vi "Velociprobe_Nanopositioner_Control_FPGA.vi"() -> ()   [LabVIEW 2015]
uses:
  <vilib>/Platform/TimedLoop/XDataNode/timing_clust.ctl
  <vilib>/Platform/TimedLoop/XDataNode/nitl_modes.ctl
  <vilib>/Platform/TimedLoop/XDataNode/wakeup.ctl
  Control X Up Down Ramp.ctl
  Control Y Up Down Ramp.ctl
  Detector_Trigger_Control.ctl
  <vilib>/rvi/Emulation/niFpgaSctlEmulationGetInTimedLoop.vi
  <vilib>/rvi/Emulation/niFpgaProcessEmulError.vi
  <vilib>/rvi/eio/common/nirviEmuTemplateMethod_errors.vi
  <vilib>/rvi/Emulation/niFpgaGetClockAttributes.vi
  <vilib>/rvi/Emulation/niFpgaEmulationReportErrorSimple.vi
  <vilib>/rvi/interface/RandomDataEmulation/niFpgaRandomDataHandleErrors.vi
  <vilib>/rvi/Emulation/niFpgaCriticalErrorInLSC.vi
  <vilib>/eio/EIONode/EIONode.xnode
  <vilib>/rvi/DataTransferAndStorage/Container/XNode/niFpgaContainer.xnode
  <vilib>/rvi/interface/RandomDataEmulation/nirviRandomDataFpgaReadWriteTemplate.vi
  <vilib>/rvi/Analysis/measure/butterworth/XNode/niFpgaButterworthFilter.xnode
  <vilib>/Platform/TimedLoop/XDataNode/XDataNode.xnode
  <vilib>/Platform/TimedLoop/XDataNode/XDNodeRunTimeDep.lvlib
panel:
  out "Number of Data Strings 2":i32
  out "Measured Data Trigger Time Period (Ticks)":u32
  in  "Data Trigger Time Period (uSec)":u32 caption="Detector Trigger Time Period (uSec)"
  out "Trigger for Data":fxp<+/-,58,25>
  out "Fly Scan Running":bool
  in  "Fly Scan Start":bool
  out "If True End Y Down Ramp":bool
  in  "Y Ramp Drop Size (nm)":fxp<+/-,16,16>
  out "Ramp Mid Range":bool
  out "If True End Up Ramp":bool
  out "Start or middle":bool=TRUE
  in  "Y Start Marker (nm)":fxp<+/-,58,25> format="%#_55g"
  out "Y Ramp Slope":fxp<+,48,16>
  in  "Y Ramp End (nm)":fxp<+/-,16,16>
  in  "Y Ramp Start (nm)":fxp<+/-,16,16>
  in  "Y Ramp Period (usec)":fxp<+,32,32>
  in  "X Ramp Period (usec)":fxp<+,32,32>
  in  "X Ramp End (nm)":fxp<+/-,16,16>
  in  "X Ramp Start (nm)":fxp<+/-,16,16>
  out "If True End X Down Ramp":bool
  out "X Ramp Mid Range":bool
  out "If True End X Up Ramp":bool
  out "Y Ramp Drop":bool
  out "Next Do Down Ramp":bool
  out "Continue Run":bool
  in  "X Start Marker (nm)":fxp<+/-,58,25>
  out "X Ramp Slope":fxp<+,48,16> format="%.37g"
  in  "DT Reset":bool
  in  "DT Duty Cycle (periods)":fxp<+,32,0>=0.5 caption="DT duty cycle (periods)"
  in  "DT Reference DC Offset (V)":fxp<+/-,16,16>
  in  "DT Reference Amplitude (V)":fxp<+/-,40,17>
  in  "DT Phase Offset (periods)":fxp<+,32,0>
  in  "DT Frequency (periods/tick)":fxp<+,32,0>=0.0002500000409781933
  in  "Trigger Wave Generator":T1(ring)
  out "If True End Trigger Low":bool
  in  "Trigger Low Level (V)":fxp<+/-,20,5>=-5.0
  in  "Trigger High Level (V)":fxp<+/-,20,5>=5.0
  out "If True End Trigger High":bool
  out "Trigger Mid High":bool
  in  "Trigger Low Period (usec)":fxp<+/-,64,45>
  in  "Trigger High Period (usec)":fxp<+/-,64,45>
  out "Measured Z Reference Time Period (Ticks)":u32
  in  "Z Reference Time Period (uSec)":u32
  in  "Z White Noise Amplitude":u16=32767
  in  "Z White Noise Seed":u32=4
  in  "Z Phase Offset (periods)":fxp<+,32,0>
  in  "Z Frequency (periods/tick)":fxp<+,32,0>=0.0002500000409781933
  in  "Z Reference DC Offset (nm)":fxp<+/-,16,16>
  in  "Z Reference Amplitude (nm)":fxp<+/-,40,17>
  in  "Z Reference Reset":bool
  in  "Z Reference Wave Selection":T2(ring)
  in  "Y White Noise Amplitude":u16=32767
  in  "Y White Noise Seed":u32=4
  out "Measured Y Reference Time Period (Ticks)":u32
  in  "Y Reference Time Period (uSec)":u32
  in  "Y Reference Reset":bool
  in  "Y Reference Wave Selection":T3(ring)
  in  "Detector Trigger Lower Limit (V)":fxp<+/-,20,5>=-5.0
  out "Detector Trigger In Range?":bool
  in  "Detector Trigger Upper Limit (V)":fxp<+/-,20,5>=5.0
  out "Detector Trigger (V)":fxp<+/-,20,5> format="%.29g"
  out "Measured Detector Trigger Time Period (Ticks)":u32
  in  "Detector Trigger Time Period (uSec)":u32
  out "Measured Trigger Gen Time Period (Ticks)":u32
  in  "Trigger Generation Time Period (uSec)":u32
  in  "Reference Signal Source":T4(ring)
  in  "Z-Stage Scaling Direction":fxp<+/-,3,3>=-1.0
  in  "Y-Stage Scaling Direction":fxp<+/-,3,3>=-1.0
  in  "Y Phase Offset (periods)":fxp<+,32,0>
  in  "Y Frequency (periods/tick)":fxp<+,32,0>=0.0002500000409781933
  in  "Optics and or Sample Stage":T5(ring)
  out "Z Stage External Reference (nm)":fxp<+/-,58,25>
  in  "Mod 3 AI2 V to nm Scaling":fxp<+,47,18>
  out "Mod 8 Input AI2 (V)":fxp<+/-,24,5>
  out "Y Stage External Reference (nm)":fxp<+/-,58,25>
  in  "Mod 3 AI1 V to nm Scaling":fxp<+,47,18>
  out "Mod 8 Input AI1 (V)":fxp<+/-,24,5>
  in  "Sample Z Stage Resolution (nm)":fxp<+,33,3>=0.001000046730041504
  in  "Sample Y Stage Resolution (nm)":fxp<+,33,3>=0.001000046730041504
  in  "Sample X Stage Resolution (nm)":fxp<+,33,3>=0.001000046730041504
  out "Sample Z Stage Displacement (nm)":fxp<+/-,58,25>
  out "Sample Z Stage Displacement raw (nm)":fxp<+/-,64,35> format="%.62g"
  out "Sample Y Stage Displacement (nm)":fxp<+/-,58,25>
  out "Sample Y Stage Displacement raw (nm)":fxp<+/-,64,35> format="%.41g"
  out "Sample X Stage Displacement raw (nm)":fxp<+/-,64,35> format="%.62g"
  out "Sample X Stage Displacement (nm)":fxp<+/-,58,25>
  in  "Reset Sample Z":bool
  out "32 bit Count Sample  Z":i32
  in  "Reset Sample Y":bool
  out "32 bit Count Sample  Y":i32
  in  "Reset Sample X":bool
  out "32 bit Count Sample X":i32
  out "Mod6/DIO3":bool
  out "Mod6/DIO2":bool
  out "Mod5/DIO3":bool
  out "Mod5/DIO2":bool
  out "Mod4/DIO3":bool
  out "Mod4/DIO2":bool
  out "Measured Analog Input Time Period (Ticks)":u32
  in  "Analog Input Time Period (uSec)":u32
  out "X Stage External Reference (nm)":fxp<+/-,58,25>
  in  "Mod 3 AI0 V to nm Scaling":fxp<+,47,18>
  out "Mod 3 Input AI0 (V)":fxp<+/-,24,5>
  out "Kxz Output, Kxz*ex (V)":fxp<+/-,58,25> format="%.31g"
  out "Kyz Output, Kyz*ey (V)":fxp<+/-,58,25> format="%.31g"
  in  "b02(2) yz1":fxp<+/-,64,9>[](array[numeric])=[0.0, 0.0, 0.0, 0.0, 0.0, 0.0, 0.0, 0.0, 0.0, 0.0, 0.0, 0.0, 0.0, 0.0, 0.0, 0.0, 0.0, 0.0, 0.0, 0.0]
  in  "b01(2) yz1":fxp<+/-,64,9>[](array[numeric])=[0.0, 0.0, 0.0, 0.0, 0.0, 0.0, 0.0, 0.0, 0.0, 0.0, 0.0, 0.0, 0.0, 0.0, 0.0, 0.0, 0.0, 0.0, 0.0, 0.0]
  in  "-a02(2) yz1":fxp<+/-,64,9>[](array[numeric])=[0.0, 0.0, 0.0, 0.0, 0.0, 0.0, 0.0, 0.0, 0.0, 0.0, 0.0, 0.0, 0.0, 0.0, 0.0, 0.0, 0.0, 0.0, 0.0, 0.0]
  in  "-a01(2) yz1":fxp<+/-,64,9>[](array[numeric])=[0.0, 0.0, 0.0, 0.0, 0.0, 0.0, 0.0, 0.0, 0.0, 0.0, 0.0, 0.0, 0.0, 0.0, 0.0, 0.0, 0.0, 0.0, 0.0, 0.0]
  in  "sos gain SF Controller yz1":fxp<+/-,42,9>
  in  "b02(2) xz1":fxp<+/-,64,9>[](array[numeric])=[0.0, 0.0, 0.0, 0.0, 0.0, 0.0, 0.0, 0.0, 0.0, 0.0, 0.0, 0.0, 0.0, 0.0, 0.0, 0.0, 0.0, 0.0, 0.0, 0.0]
  in  "b01(2) xz1":fxp<+/-,64,9>[](array[numeric])=[0.0, 0.0, 0.0, 0.0, 0.0, 0.0, 0.0, 0.0, 0.0, 0.0, 0.0, 0.0, 0.0, 0.0, 0.0, 0.0, 0.0, 0.0, 0.0, 0.0]
  in  "-a02(2) xz1":fxp<+/-,64,9>[](array[numeric])=[0.0, 0.0, 0.0, 0.0, 0.0, 0.0, 0.0, 0.0, 0.0, 0.0, 0.0, 0.0, 0.0, 0.0, 0.0, 0.0, 0.0, 0.0, 0.0, 0.0]
  in  "-a01(2) xz1":fxp<+/-,64,9>[](array[numeric])=[0.0, 0.0, 0.0, 0.0, 0.0, 0.0, 0.0, 0.0, 0.0, 0.0, 0.0, 0.0, 0.0, 0.0, 0.0, 0.0, 0.0, 0.0, 0.0, 0.0]
  in  "sos gain SF Controller xz1":fxp<+/-,42,9>
  out "Kzy Output, Kzy*ez (V)":fxp<+/-,58,25> format="%.31g"
  out "Kxy Output, Kxy*ex (V)":fxp<+/-,58,25> format="%.31g"
  in  "b02(2) zy1":fxp<+/-,64,9>[](array[numeric])=[0.0, 0.0, 0.0, 0.0, 0.0, 0.0, 0.0, 0.0, 0.0, 0.0, 0.0, 0.0, 0.0, 0.0, 0.0, 0.0, 0.0, 0.0, 0.0, 0.0]
  in  "b01(2) zy1":fxp<+/-,64,9>[](array[numeric])=[0.0, 0.0, 0.0, 0.0, 0.0, 0.0, 0.0, 0.0, 0.0, 0.0, 0.0, 0.0, 0.0, 0.0, 0.0, 0.0, 0.0, 0.0, 0.0, 0.0]
  in  "-a02(2) zy1":fxp<+/-,64,9>[](array[numeric])=[0.0, 0.0, 0.0, 0.0, 0.0, 0.0, 0.0, 0.0, 0.0, 0.0, 0.0, 0.0, 0.0, 0.0, 0.0, 0.0, 0.0, 0.0, 0.0, 0.0]
  in  "-a01(2) zy1":fxp<+/-,64,9>[](array[numeric])=[0.0, 0.0, 0.0, 0.0, 0.0, 0.0, 0.0, 0.0, 0.0, 0.0, 0.0, 0.0, 0.0, 0.0, 0.0, 0.0, 0.0, 0.0, 0.0, 0.0]
  in  "sos gain SF Controller zy1":fxp<+/-,42,9>
  in  "b02(2) xy1":fxp<+/-,64,9>[](array[numeric])=[0.0, 0.0, 0.0, 0.0, 0.0, 0.0, 0.0, 0.0, 0.0, 0.0, 0.0, 0.0, 0.0, 0.0, 0.0, 0.0, 0.0, 0.0, 0.0, 0.0]
  in  "b01(2) xy1":fxp<+/-,64,9>[](array[numeric])=[0.0, 0.0, 0.0, 0.0, 0.0, 0.0, 0.0, 0.0, 0.0, 0.0, 0.0, 0.0, 0.0, 0.0, 0.0, 0.0, 0.0, 0.0, 0.0, 0.0]
  in  "-a02(2) xy1":fxp<+/-,64,9>[](array[numeric])=[0.0, 0.0, 0.0, 0.0, 0.0, 0.0, 0.0, 0.0, 0.0, 0.0, 0.0, 0.0, 0.0, 0.0, 0.0, 0.0, 0.0, 0.0, 0.0, 0.0]
  in  "-a01(2) xy1":fxp<+/-,64,9>[](array[numeric])=[0.0, 0.0, 0.0, 0.0, 0.0, 0.0, 0.0, 0.0, 0.0, 0.0, 0.0, 0.0, 0.0, 0.0, 0.0, 0.0, 0.0, 0.0, 0.0, 0.0]
  in  "sos gain SF Controller xy1":fxp<+/-,42,9>
  out "Kzx Output, Kzx*ez (V)":fxp<+/-,58,25> format="%.31g"
  in  "b02(2) zx1":fxp<+/-,64,9>[](array[numeric])=[0.0, 0.0, 0.0, 0.0, 0.0, 0.0, 0.0, 0.0, 0.0, 0.0, 0.0, 0.0, 0.0, 0.0, 0.0, 0.0, 0.0, 0.0, 0.0, 0.0]
  in  "b01(2) zx1":fxp<+/-,64,9>[](array[numeric])=[0.0, 0.0, 0.0, 0.0, 0.0, 0.0, 0.0, 0.0, 0.0, 0.0, 0.0, 0.0, 0.0, 0.0, 0.0, 0.0, 0.0, 0.0, 0.0, 0.0]
  in  "-a02(2) zx1":fxp<+/-,64,9>[](array[numeric])=[0.0, 0.0, 0.0, 0.0, 0.0, 0.0, 0.0, 0.0, 0.0, 0.0, 0.0, 0.0, 0.0, 0.0, 0.0, 0.0, 0.0, 0.0, 0.0, 0.0]
  in  "-a01(2) zx1":fxp<+/-,64,9>[](array[numeric])=[0.0, 0.0, 0.0, 0.0, 0.0, 0.0, 0.0, 0.0, 0.0, 0.0, 0.0, 0.0, 0.0, 0.0, 0.0, 0.0, 0.0, 0.0, 0.0, 0.0]
  in  "sos gain SF Controller zx1":fxp<+/-,42,9>
  out "Kyx Output, Kyx*ey (V)":fxp<+/-,58,25> format="%.31g"
  in  "b02(2) yx1":fxp<+/-,64,9>[](array[numeric])=[0.0, 0.0, 0.0, 0.0, 0.0, 0.0, 0.0, 0.0, 0.0, 0.0, 0.0, 0.0, 0.0, 0.0, 0.0, 0.0, 0.0, 0.0, 0.0, 0.0]
  in  "b01(2) yx1":fxp<+/-,64,9>[](array[numeric])=[0.0, 0.0, 0.0, 0.0, 0.0, 0.0, 0.0, 0.0, 0.0, 0.0, 0.0, 0.0, 0.0, 0.0, 0.0, 0.0, 0.0, 0.0, 0.0, 0.0]
  in  "-a02(2) yx1":fxp<+/-,64,9>[](array[numeric])=[0.0, 0.0, 0.0, 0.0, 0.0, 0.0, 0.0, 0.0, 0.0, 0.0, 0.0, 0.0, 0.0, 0.0, 0.0, 0.0, 0.0, 0.0, 0.0, 0.0]
  in  "-a01(2) yx1":fxp<+/-,64,9>[](array[numeric])=[0.0, 0.0, 0.0, 0.0, 0.0, 0.0, 0.0, 0.0, 0.0, 0.0, 0.0, 0.0, 0.0, 0.0, 0.0, 0.0, 0.0, 0.0, 0.0, 0.0]
  in  "sos gain SF Controller yx1":fxp<+/-,42,9>
  in  "X-Stage Scaling Direction":fxp<+/-,3,3>=-1.0
  in  "Z-Stage nm to V Scaling":fxp<+/-,32,12>
  in  "Y-Stage nm to V Scaling":fxp<+/-,32,12>
  in  "X-Stage nm to V Scaling":fxp<+/-,32,12>
  out "Kxx Output, Kxx*ex (V)":fxp<+/-,58,25>
  out "Kyy Output, Kyy*ey (V)":fxp<+/-,58,25>
  out "Kzz Output, Kzz*ez (V)":fxp<+/-,58,25>
  in  "sos gain SF Controller xx1":fxp<+/-,42,9>
  in  "-a01(2) xx1":fxp<+/-,64,9>[](array[numeric])=[0.0, 0.0, 0.0, 0.0, 0.0, 0.0, 0.0, 0.0, 0.0, 0.0, 0.0, 0.0, 0.0, 0.0, 0.0, 0.0, 0.0, 0.0, 0.0, 0.0]
  in  "-a02(2) xx1":fxp<+/-,64,9>[](array[numeric])=[0.0, 0.0, 0.0, 0.0, 0.0, 0.0, 0.0, 0.0, 0.0, 0.0, 0.0, 0.0, 0.0, 0.0, 0.0, 0.0, 0.0, 0.0, 0.0, 0.0]
  in  "b01(2) xx1":fxp<+/-,64,9>[](array[numeric])=[0.0, 0.0, 0.0, 0.0, 0.0, 0.0, 0.0, 0.0, 0.0, 0.0, 0.0, 0.0, 0.0, 0.0, 0.0, 0.0, 0.0, 0.0, 0.0, 0.0]
  in  "b02(2) xx1":fxp<+/-,64,9>[](array[numeric])=[0.0, 0.0, 0.0, 0.0, 0.0, 0.0, 0.0, 0.0, 0.0, 0.0, 0.0, 0.0, 0.0, 0.0, 0.0, 0.0, 0.0, 0.0, 0.0, 0.0]
  in  "sos gain SF Controller yy1":fxp<+/-,42,9>
  in  "-a01(2) yy1":fxp<+/-,64,9>[](array[numeric])=[0.0, 0.0, 0.0, 0.0, 0.0, 0.0, 0.0, 0.0, 0.0, 0.0, 0.0, 0.0, 0.0, 0.0, 0.0, 0.0, 0.0, 0.0, 0.0, 0.0]
  in  "-a02(2) yy1":fxp<+/-,64,9>[](array[numeric])=[0.0, 0.0, 0.0, 0.0, 0.0, 0.0, 0.0, 0.0, 0.0, 0.0, 0.0, 0.0, 0.0, 0.0, 0.0, 0.0, 0.0, 0.0, 0.0, 0.0]
  in  "b01(2) yy1":fxp<+/-,64,9>[](array[numeric])=[0.0, 0.0, 0.0, 0.0, 0.0, 0.0, 0.0, 0.0, 0.0, 0.0, 0.0, 0.0, 0.0, 0.0, 0.0, 0.0, 0.0, 0.0, 0.0, 0.0]
  in  "b02(2) yy1":fxp<+/-,64,9>[](array[numeric])=[0.0, 0.0, 0.0, 0.0, 0.0, 0.0, 0.0, 0.0, 0.0, 0.0, 0.0, 0.0, 0.0, 0.0, 0.0, 0.0, 0.0, 0.0, 0.0, 0.0]
  in  "sos gain SF Controller zz1":fxp<+/-,42,9>
  in  "-a01(2) zz1":fxp<+/-,64,9>[](array[numeric])=[0.0, 0.0, 0.0, 0.0, 0.0, 0.0, 0.0, 0.0, 0.0, 0.0, 0.0, 0.0, 0.0, 0.0, 0.0, 0.0, 0.0, 0.0, 0.0, 0.0]
  in  "-a02(2) zz1":fxp<+/-,64,9>[](array[numeric])=[0.0, 0.0, 0.0, 0.0, 0.0, 0.0, 0.0, 0.0, 0.0, 0.0, 0.0, 0.0, 0.0, 0.0, 0.0, 0.0, 0.0, 0.0, 0.0, 0.0]
  in  "b01(2) zz1":fxp<+/-,64,9>[](array[numeric])=[0.0, 0.0, 0.0, 0.0, 0.0, 0.0, 0.0, 0.0, 0.0, 0.0, 0.0, 0.0, 0.0, 0.0, 0.0, 0.0, 0.0, 0.0, 0.0, 0.0]
  in  "b02(2) zz1":fxp<+/-,64,9>[](array[numeric])=[0.0, 0.0, 0.0, 0.0, 0.0, 0.0, 0.0, 0.0, 0.0, 0.0, 0.0, 0.0, 0.0, 0.0, 0.0, 0.0, 0.0, 0.0, 0.0, 0.0]
  in  "Scaling mV to V":fxp<+,33,10>=0.0009765625
  in  "System Loop Type":enum16{"Open Loop", "Closed Loop"}(ring)
  in  "Timeout FPGA FIFO1":i32=40000000
  out "FIFO Timed Out":bool
  in  "Interrupt Boolean":bool
  out "Wait Until Cleared":bool
  out "Number of Data Strings":i32
  in  "Y Reference DC Offset (nm)":fxp<+/-,16,16>
  in  "X Reference DC Offset (nm)":fxp<+/-,16,16>
  in  "Y Reference Amplitude (nm)":fxp<+/-,40,17>
  out "Z Stage Reference (nm)":fxp<+/-,58,25> format="%.41g"
  out "Y Stage Reference (nm)":fxp<+/-,58,25> format="%.41g"
  out "Optics Z Stage Displacement (nm)":fxp<+/-,58,25>
  out "Optics Z Stage Displacement raw (nm)":fxp<+/-,64,35>
  in  "Optics Z Stage Resolution (nm)":fxp<+,33,3>=0.001000046730041504
  in  "Reset Optics Z":bool
  out "32 bit Count Optics  Z":i32
  out "Mod6/DIO1":bool
  out "Mod6/DIO0":bool
  out "Optics Y Stage Displacement (nm)":fxp<+/-,58,25>
  out "Optics Y Stage Displacement raw (nm)":fxp<+/-,64,35>
  in  "Optics Y Stage Resolution (nm)":fxp<+,33,3>=0.001000046730041504
  in  "Reset Optics Y":bool
  out "32 bit Count Optics  Y":i32
  out "Mod5/DIO1":bool
  out "Mod5/DIO0":bool
  out "Z-Stage Input In Range?":bool
  out "Y-Stage Input In Range?":bool
  in  "Controller Output Lower Limit":fxp<+/-,20,5>=-5.0
  out "X-Stage Input In Range?":bool
  in  "Controller Output Upper Limit":fxp<+/-,20,5>=5.0
  in  "X White Noise Amplitude":u16=32767
  in  "X White Noise Seed":u32=4
  in  "X Reference Reset":bool
  in  "X Reference Wave Selection":T6(ring)
  out "Measured Counter Time Period (Ticks)":u32
  out "Measured Datalog Time Period (Ticks)":u32
  out "Measured Plant Output Time Period (Ticks)":u32
  out "Measured Controller Output Time Period (Ticks)":u32
  out "Measured Controller Time Period (Ticks)":u32
  out "Measured X Reference Time Period (Ticks)":u32
  out "Optics X Stage Displacement raw (nm)":fxp<+/-,64,35>
  in  "Optics X Stage Resolution (nm)":fxp<+,33,3>=0.001000046730041504 format="%#_31g"
  in  "Plant Output Time Period (uSec)":u32
  out "Optics X Stage Displacement (nm)":fxp<+/-,58,25>
  in  "Reset Optics X":bool
  out "32 bit Count Optics X":i32
  out "Mod4/DIO1":bool
  out "Mod4/DIO0":bool
  out "error out (FPGA)":errorcluster
  out "error out (AO FPGA)":errorcluster
  out "stop case":bool
  in  "Controller Output Time Period (uSec)":u32
  in  "Datalog Cases":T7(ring)
  out "PI Z-Stage Input (V)":fxp<+/-,20,5> format="%.29g"
  out "PI Y-Stage Input (V)":fxp<+/-,20,5> format="%.29g"
  out "PI X-Stage Input (V)":fxp<+/-,20,5> format="%.29g"
  in  "Controller Time Period (uSec)":u32
  in  "Datalog Time Period (uSec)":u32
  in  "X Reference Time Period (uSec)":u32
  in  "X Reference Amplitude (nm)":fxp<+/-,40,17>
  out "X Stage Reference (nm)":fxp<+/-,58,25> format="%.41g"
  out "FIFO Timed Out?":bool
  in  "X Phase Offset (periods)":fxp<+,32,0>
  in  "X Frequency (periods/tick)":fxp<+,32,0>=0.0002500000409781933
types:
  T1 = enum16{"Custom Square Wave ", "Square Wave 1", "Square Wave 2"}
  T2 = enum16{"Constant", "Sine Wave", "Sawtooth Wave", "Square Wave", "Filtered White Noise"}
  T3 = enum16{"Constant", "Sine Wave", "Custom Ramp Wave", "Filtered White Noise"}
  T4 = enum16{"FPGA Generated Reference", "External Reference"}
  T5 = enum16{"Optics Stage Only", "Optics and Sample Stage"}
  T6 = enum16{"Constant", "Sine Wave", "Custom Up Down Ramp", "Filtered White Noise"}
  T7 = enum16{"Data Log 1", "Data Log 2", "Data Log 3", "Data Log 4", "Data Log 5", "Data Log 6", "Data Log 7", "Data Log 8", "Data Log 9", "Data Log 10", "Data Log 11", "Data Log 12", "Data Log 13", "Data Log 14", "Data Log 15", "Data Log 16"}
  T8 = typedef "Control Y Up Down Ramp.ctl" = enum16{"Y Up Ramp", "Y Down Ramp"}
  T9 = typedef "Detector_Trigger_Control.ctl" = enum16{"Trigger High", "Trigger Low"}
  T10 = typedef "XDNodeRunTimeDep.lvlib/timing_clust.ctl" = cluster{"Expected End [f-1]":u64, "Actual End [f-1]":u64, "Finished Late? [f-1]":bool, "Expected End [i-1]":u64, "Actual End [i-1]":u64, "Finished Late? [i-1]":bool, "Expected Start [i]":u64, "Actual Start [i]":u64, "Expected Start [f]":u64, "Actual Start [f]":u64, "Source Name":string, "Structure Name":string, "Period":i64, "Deadline":i64, "Offset":i64, "Start":i64, "Priority":i32, "Timeout":i32, "Mode":T11, "Wakeup Reason":T12, "Error":errorcluster, "Source Type":string, "Secondary Source Type":string, "Global End Time":u64, "Global Start Time":u64, "Frame Duration":u64, "Iteration Duration":u64, "Assigned CPU":i32, "I/O Scan Engine Mode":u32}
  T11 = typedef "XDNodeRunTimeDep.lvlib/nitl_modes.ctl" = enum32{"No Change", "Process missed periods, maintain original phase", "Discard missed periods, maintain original phase", "Process missed periods, ignore original phase", "Discard missed periods, ignore original phase"}
  T12 = typedef "XDNodeRunTimeDep.lvlib/wakeup.ctl" = enum32{"Normal", "Aborted", "Asynchronous wakeup", "Timing source error", "Timed loop error", "Timeout"}
  T13 = typedef "Control X Up Down Ramp.ctl" = enum16{"X Up Ramp", "X Down Ramp"}
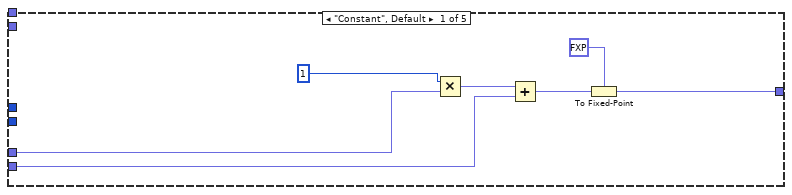
[diagram p2: hidden frame]
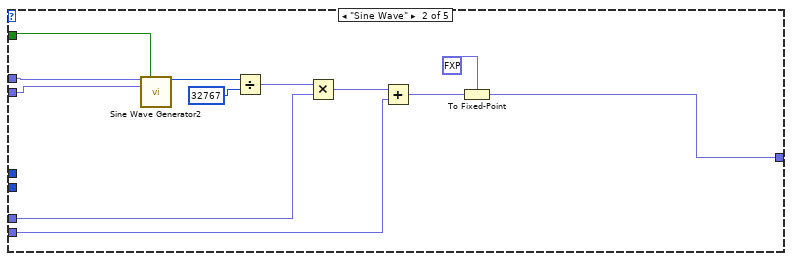
[diagram p3: hidden frame]
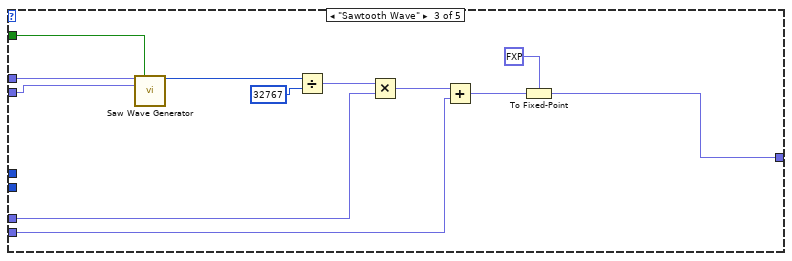
[diagram p4: hidden frame]
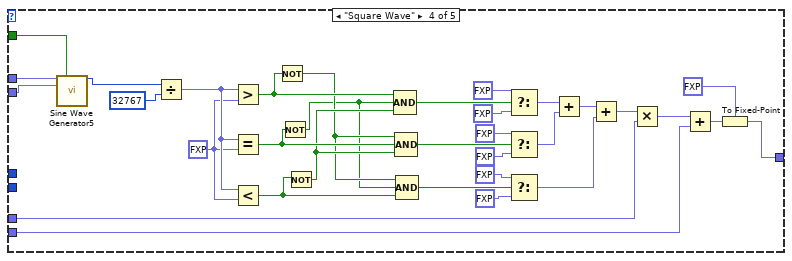
[diagram p5: hidden frame]
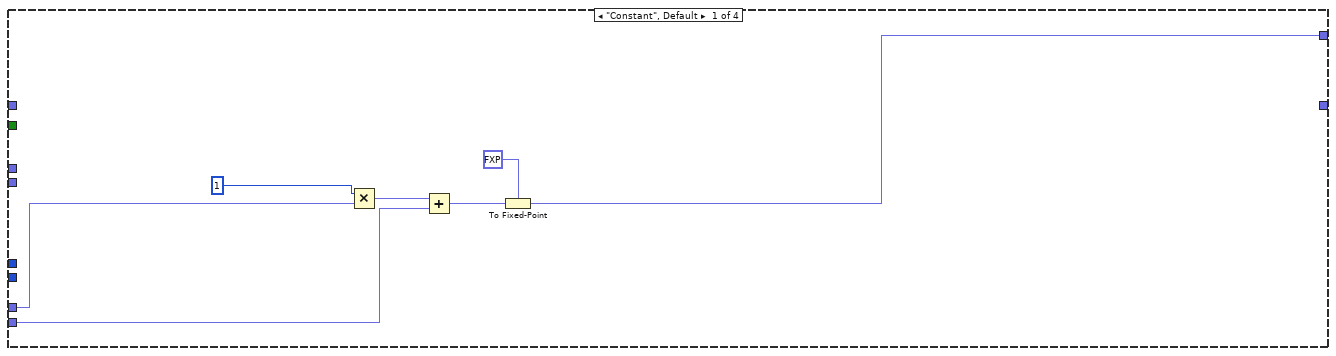
[diagram p6: hidden frame]
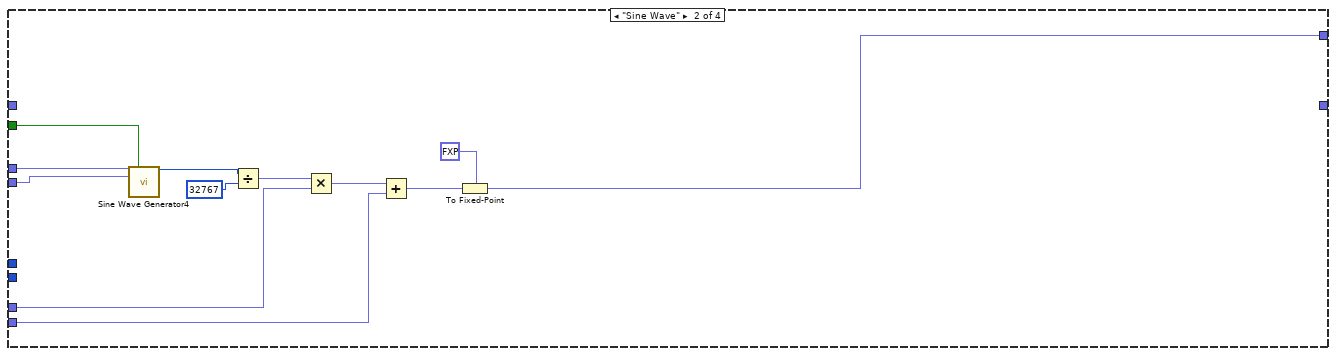
[diagram p7: hidden frame]
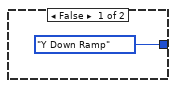
[diagram p8: hidden frame]
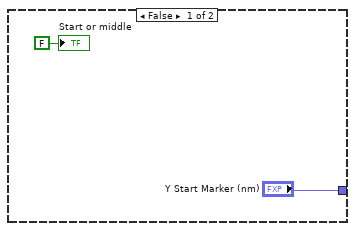
[diagram p9: hidden frame]
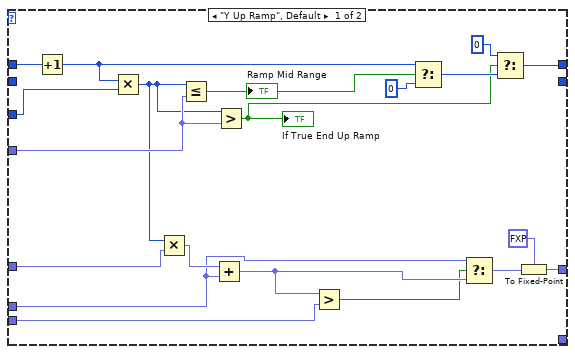
[diagram p10: hidden frame]
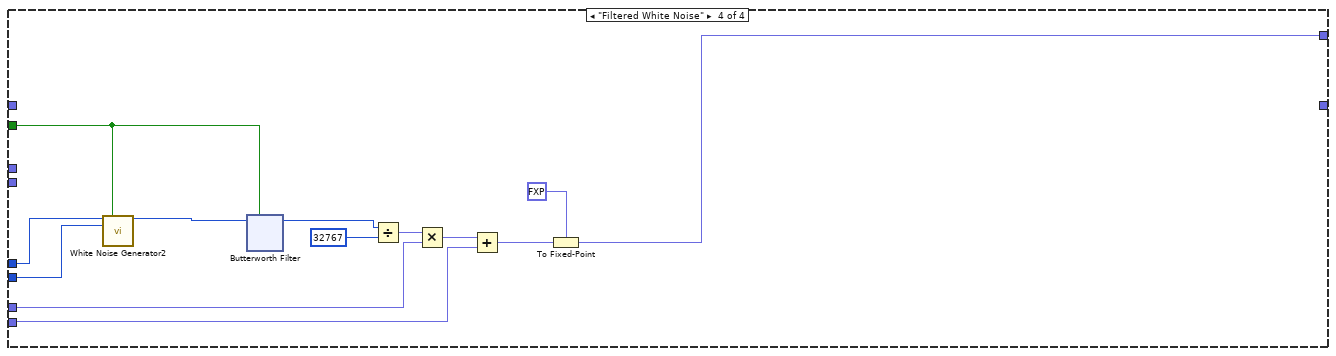
[diagram p13: hidden frame]
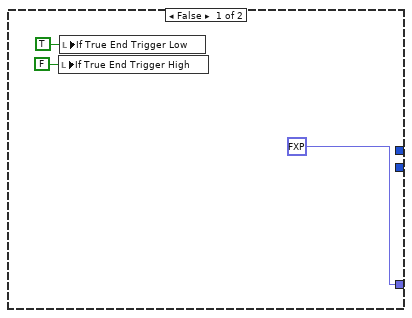
[diagram p14: hidden frame]
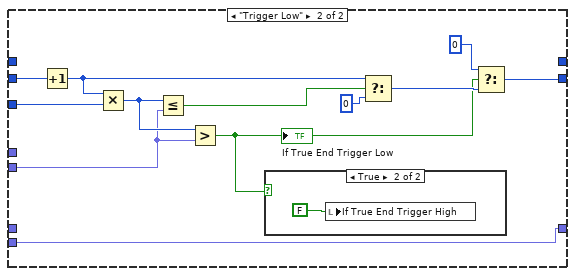
[diagram p16: hidden frame]
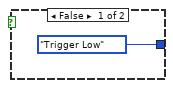
[diagram p18: hidden frame]
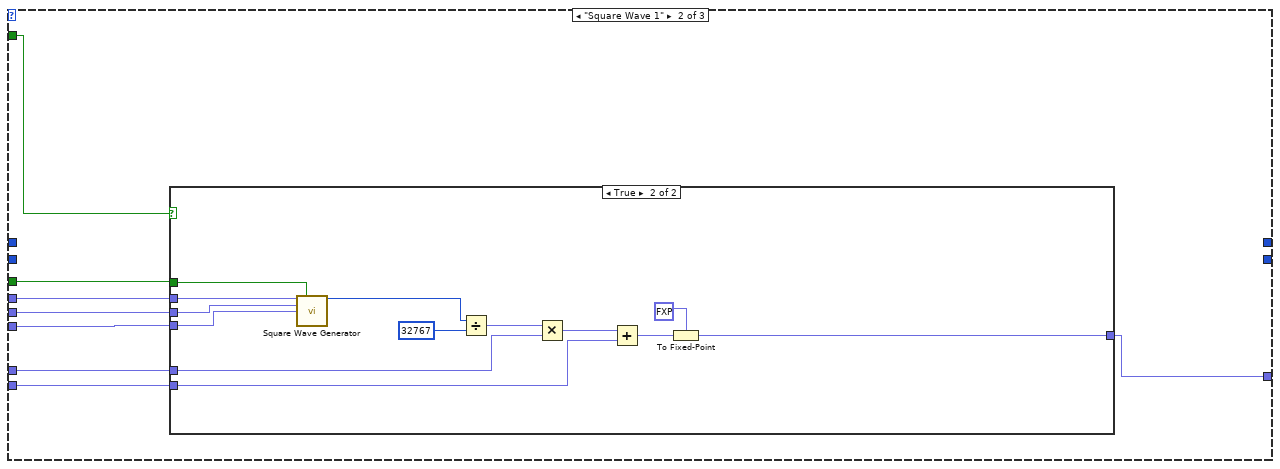
[diagram p19: hidden frame]
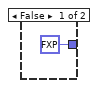
[diagram p20: hidden frame]
diagram:
  n1 = flat-sequence {
    tunnel: [w4] -> w1
    tunnel: [w10] -> w3
    tunnel: w1 -> [w10]
    frame #0 {
      n2 = xnode "FPGA I/O Node"("Mod3/Start"=TRUE ("I/O Item")) -> ("error out"=w4:errorcluster)  [unwired: 2 in, 1 out]
      "error out (AO FPGA)" <- w4
      "stop case" <- FALSE ("stop case")
    }
    frame #1 {
      w9 = u8 0  # IRQ Number (0)
      n3 = Not(x="Interrupt Boolean") -> (.not. x?=w7:bool)
      "Wait Until Cleared" <- w7
      n4 = call <vilib>:"niFPGA Interrupt.vi"("Wait Until Cleared (F)"=w7, "IRQ Number (0)"=w9) -> ()  [unwired: 1 in]
    }
  }
  n5 = case shown="No Error" w3 {
    selector: w3 -> [_ w1943]
    tunnel: [w30 w1943] -> w2
    frame No Error {
      w21 = errorcluster {"status"=FALSE, "code"=0, "source"=""}  # Error
      w15 = 0
      n6 = while {
        tunnel: [w1554] -> w24
        shift-right: [w1547] -> _
        shift-left: _ -> [w1546]
        shift-right: [w1543] -> _
        shift-left: _ -> [w1542]
        stop <- w1552 stop-if-true
        n7 = local read "Detector Trigger (V)"() -> (w1547:fxp<+/-,20,5>)
        n8 = local read "Trigger for Data"() -> (w1543:fxp<+/-,58,25>)
        n9 = local read "Fly Scan Running"() -> (w1544:bool)
        n10 = Greater?(x=w1547, y=w1546) -> (0:w1545:bool)
        n11 = Greater?(x=w1543, y=w1542) -> (0:w1541:bool)
        n12 = case shown="True" w1544 {
          tunnel: [w1558 w1571] -> w1555
          tunnel: [w1559 w1570] -> w1548
          tunnel: w1545 -> [_ w1569]
          tunnel: w1541 -> [w1557 _]
          frame False {
            w1566 = 5  # # of Data Strings
            n13 = case shown="True" w1557 {
              tunnel: w1566 -> [_ w1567]
              tunnel: fxp<+/-,58,25> 0.0 ("fixed-point type") -> [_ w1568]
              tunnel: [_ w1568] -> w1564
              tunnel: [_ w1568] -> w1562
              tunnel: [_ w1568] -> w1561
              tunnel: [_ w1568] -> w1560
              tunnel: [_ w1568] -> w1563
              tunnel: [_ w1567] -> w1558
              frame False {
              }
              frame True {
              }
            }
            "Number of Data Strings 2" <- w1558
            n14 = Build Array "Build Array"(w1564, w1563, w1562, w1561, w1560) -> (w1559:fxp<+/-,58,25>[])
          }
          frame True {
            n15 = case shown="True" w1569 {
              tunnel: [_ w1578] -> w1571
              tunnel: [_ w1574] -> w1570
              frame False {
              }
              frame True {
                w1579 = 5  # # of Data Strings
                n16 = local read "Sample X Stage Displacement (nm)"() -> (w1585:fxp<+/-,58,25>)
                n17 = local read "Sample Y Stage Displacement (nm)"() -> (w1584:fxp<+/-,58,25>)
                n18 = local read "Sample Z Stage Displacement (nm)"() -> (w1583:fxp<+/-,58,25>)
                n19 = local read "Optics X Stage Displacement (nm)"() -> (w1589:fxp<+/-,58,25>)
                n20 = local read "Optics Y Stage Displacement (nm)"() -> (w1588:fxp<+/-,58,25>)
                n21 = local read "Optics Z Stage Displacement (nm)"() -> (w1586:fxp<+/-,58,25>)
                n22 = local read "X Stage External Reference (nm)"() -> (w1577:fxp<+/-,58,25>)
                n23 = local read "Y Stage External Reference (nm)"() -> (w1576:fxp<+/-,58,25>)
                n24 = local read "Z Stage External Reference (nm)"() -> (w1575:fxp<+/-,58,25>)
                n25 = local read "X Stage Reference (nm)"() -> (w1597:fxp<+/-,58,25>)
                n26 = local read "Y Stage Reference (nm)"() -> (w1582:fxp<+/-,58,25>)
                n27 = local read "Z Stage Reference (nm)"() -> (w1581:fxp<+/-,58,25>)
                n28 = local read "Detector Trigger (V)"() -> (w1573:fxp<+/-,20,5>)
                n29 = local read "PI X-Stage Input (V)"() -> (w1596:fxp<+/-,20,5>)
                n30 = local read "PI Y-Stage Input (V)"() -> (w1595:fxp<+/-,20,5>)
                n31 = local read "PI Z-Stage Input (V)"() -> (w1594:fxp<+/-,20,5>)
                n32 = case shown="\"Data Log 16\"" "Datalog Cases" {
                  tunnel: fxp<+/-,58,25> 0.0 ("fixed-point type") -> [w1599 w1612 w1621 w1634 w1643 w1658 w1671 w1683 w1701 w1713 w1723 w1735 w1746 w1758 w1769 w1781]
                  tunnel: [w1608 w1619 w1631 w1642 w1655 w1668 w1678 w1695 w1705 w1719 w1728 w1743 w1755 w1766 w1777 w1789] -> w1592
                  tunnel: w1597 -> [w1609 _ _ _ w1648 _ _ _ _ _ _ _ _ _ _ w1785]
                  tunnel: w1596 -> [w1605 _ _ _ w1647 _ _ _ _ w1720 _ _ w1750 _ _ _]
                  tunnel: w1595 -> [_ w1618 _ _ _ w1662 _ _ _ _ w1733 _ _ w1761 _ _]
                  tunnel: w1594 -> [_ _ w1628 _ _ _ w1675 _ _ _ _ w1744 _ _ w1772 _]
                  tunnel: [w1607 w1611 w1630 w1636 w1654 w1667 w1677 w1691 w1704 w1714 w1727 w1742 w1754 w1765 w1776 w1788] -> w1591
                  tunnel: [w1606 w1620 w1629 w1641 w1653 w1666 w1676 w1687 w1703 w1715 w1726 w1741 w1753 w1764 w1775 w1787] -> w1590
                  tunnel: w1589 -> [w1602 _ _ w1638 w1650 _ _ w1698 _ w1718 w1732 w1739 w1749 _ _ w1783]
                  tunnel: w1588 -> [_ w1614 _ w1637 _ w1661 _ w1694 _ w1717 w1731 w1738 _ w1760 _ w1782]
                  tunnel: fxp<+/-,40,17> 0.0 ("fixed-point type") -> [w1601 w1613 w1623 w1632 w1645 w1657 w1669 w1682 w1699 w1710 w1722 w1734 w1748 w1757 w1768 _]
                  tunnel: w1586 -> [_ _ w1624 w1635 _ _ w1674 w1690 _ w1711 w1730 w1737 _ _ w1771 _]
                  tunnel: w1585 -> [_ _ _ _ w1649 _ _ w1697 w1708 _ _ _ _ _ _ _]
                  tunnel: w1584 -> [_ _ _ _ _ w1660 _ w1693 w1707 _ _ _ _ _ _ _]
                  tunnel: w1583 -> [_ _ _ _ _ _ w1673 w1689 w1706 _ _ _ _ _ _ _]
                  tunnel: w1582 -> [_ w1617 _ _ _ w1663 _ _ _ _ _ _ _ _ _ w1784]
                  tunnel: w1581 -> [_ _ w1627 _ _ _ w1679 _ _ _ _ _ _ _ _ _]
                  tunnel: [w1604 w1616 w1626 w1640 w1652 w1665 w1672 w1686 w1702 w1716 w1725 w1740 w1752 w1763 w1774 w1786] -> w1580
                  tunnel: w1579 -> [w1603 w1615 w1625 w1639 w1651 w1664 w1680 w1685 w1709 w1721 w1729 w1745 w1756 w1767 w1778 w1790]
                  tunnel: [w1603 w1615 w1625 w1639 w1651 w1664 w1680 w1685 w1709 w1721 w1729 w1745 w1756 w1767 w1778 w1790] -> w1578
                  tunnel: w1577 -> [_ _ _ _ _ _ _ _ _ _ _ _ w1751 _ _ _]
                  tunnel: w1576 -> [_ _ _ _ _ _ _ _ _ _ _ _ _ w1762 _ _]
                  tunnel: w1575 -> [_ _ _ _ _ _ _ _ _ _ _ _ _ _ w1773 _]
                  tunnel: w1573 -> [_ _ _ _ _ _ _ _ _ _ _ _ _ _ _ w1780]
                  tunnel: [w1600 w1610 w1622 w1633 w1644 w1656 w1670 w1684 w1700 w1712 w1724 w1736 w1747 w1759 w1770 w1779] -> w1572
                  frame "Data Log 1", Default {
                    n33 = To Fixed-Point(fixed-point type=w1599, number=w1609) -> (fixed-point=w1608:fxp<+/-,58,25>)
                    n34 = To Fixed-Point(fixed-point type=w1599, number=w1605) -> (fixed-point=w1607:fxp<+/-,58,25>)
                    n35 = To Fixed-Point(fixed-point type=w1599, number=w1602) -> (fixed-point=w1606:fxp<+/-,58,25>)
                    n36 = To Fixed-Point(fixed-point type=w1599, number=w1601) -> (fixed-point=w1604:fxp<+/-,58,25>)
                    n37 = To Fixed-Point(fixed-point type=w1599, number=w1601) -> (fixed-point=w1600:fxp<+/-,58,25>)
                  }
                  frame "Data Log 2" {
                    n38 = To Fixed-Point(fixed-point type=w1612, number=w1617) -> (fixed-point=w1619:fxp<+/-,58,25>)
                    n39 = To Fixed-Point(fixed-point type=w1612, number=w1618) -> (fixed-point=w1611:fxp<+/-,58,25>)
                    n40 = To Fixed-Point(fixed-point type=w1612, number=w1614) -> (fixed-point=w1620:fxp<+/-,58,25>)
                    n41 = To Fixed-Point(fixed-point type=w1612, number=w1613) -> (fixed-point=w1616:fxp<+/-,58,25>)
                    n42 = To Fixed-Point(fixed-point type=w1612, number=w1613) -> (fixed-point=w1610:fxp<+/-,58,25>)
                  }
                  frame "Data Log 3" {
                    n43 = To Fixed-Point(fixed-point type=w1621, number=w1627) -> (fixed-point=w1631:fxp<+/-,58,25>)
                    n44 = To Fixed-Point(fixed-point type=w1621, number=w1628) -> (fixed-point=w1630:fxp<+/-,58,25>)
                    n45 = To Fixed-Point(fixed-point type=w1621, number=w1624) -> (fixed-point=w1629:fxp<+/-,58,25>)
                    n46 = To Fixed-Point(fixed-point type=w1621, number=w1623) -> (fixed-point=w1626:fxp<+/-,58,25>)
                    n47 = To Fixed-Point(fixed-point type=w1621, number=w1623) -> (fixed-point=w1622:fxp<+/-,58,25>)
                  }
                  frame "Data Log 4" {
                    n48 = To Fixed-Point(fixed-point type=w1634, number=w1638) -> (fixed-point=w1642:fxp<+/-,58,25>)
                    n49 = To Fixed-Point(fixed-point type=w1634, number=w1637) -> (fixed-point=w1636:fxp<+/-,58,25>)
                    n50 = To Fixed-Point(fixed-point type=w1634, number=w1635) -> (fixed-point=w1641:fxp<+/-,58,25>)
                    n51 = To Fixed-Point(fixed-point type=w1634, number=w1632) -> (fixed-point=w1640:fxp<+/-,58,25>)
                    n52 = To Fixed-Point(fixed-point type=w1634, number=w1632) -> (fixed-point=w1633:fxp<+/-,58,25>)
                  }
                  frame "Data Log 5" {
                    n53 = To Fixed-Point(fixed-point type=w1643, number=w1648) -> (fixed-point=w1655:fxp<+/-,58,25>)
                    n54 = Subtract(x=w1650, y=w1649) -> (x-y=w1646:fxp<+/-,59,26>)
                    n55 = To Fixed-Point(fixed-point type=w1643, number=w1647) -> (fixed-point=w1654:fxp<+/-,58,25>)
                    n56 = To Fixed-Point(fixed-point type=w1643, number=w1646) -> (fixed-point=w1653:fxp<+/-,58,25>)
                    n57 = To Fixed-Point(fixed-point type=w1643, number=w1645) -> (fixed-point=w1652:fxp<+/-,58,25>)
                    n58 = To Fixed-Point(fixed-point type=w1643, number=w1645) -> (fixed-point=w1644:fxp<+/-,58,25>)
                  }
                  frame "Data Log 6" {
                    n59 = To Fixed-Point(fixed-point type=w1658, number=w1663) -> (fixed-point=w1668:fxp<+/-,58,25>)
                    n60 = To Fixed-Point(fixed-point type=w1658, number=w1662) -> (fixed-point=w1667:fxp<+/-,58,25>)
                    n61 = Subtract(x=w1661, y=w1660) -> (x-y=w1659:fxp<+/-,59,26>)
                    n62 = To Fixed-Point(fixed-point type=w1658, number=w1659) -> (fixed-point=w1666:fxp<+/-,58,25>)
                    n63 = To Fixed-Point(fixed-point type=w1658, number=w1657) -> (fixed-point=w1665:fxp<+/-,58,25>)
                    n64 = To Fixed-Point(fixed-point type=w1658, number=w1657) -> (fixed-point=w1656:fxp<+/-,58,25>)
                  }
                  frame "Data Log 7" {
                    n65 = To Fixed-Point(fixed-point type=w1671, number=w1679) -> (fixed-point=w1678:fxp<+/-,58,25>)
                    n66 = To Fixed-Point(fixed-point type=w1671, number=w1675) -> (fixed-point=w1677:fxp<+/-,58,25>)
                    n67 = Subtract(x=w1674, y=w1673) -> (x-y=w1681:fxp<+/-,59,26>)
                    n68 = To Fixed-Point(fixed-point type=w1671, number=w1681) -> (fixed-point=w1676:fxp<+/-,58,25>)
                    n69 = To Fixed-Point(fixed-point type=w1671, number=w1669) -> (fixed-point=w1672:fxp<+/-,58,25>)
                    n70 = To Fixed-Point(fixed-point type=w1671, number=w1669) -> (fixed-point=w1670:fxp<+/-,58,25>)
                  }
                  frame "Data Log 8" {
                    n71 = Subtract(x=w1698, y=w1697) -> (x-y=w1696:fxp<+/-,59,26>)
                    n72 = Subtract(x=w1694, y=w1693) -> (x-y=w1692:fxp<+/-,59,26>)
                    n73 = To Fixed-Point(fixed-point type=w1683, number=w1696) -> (fixed-point=w1695:fxp<+/-,58,25>)
                    n74 = Subtract(x=w1690, y=w1689) -> (x-y=w1688:fxp<+/-,59,26>)
                    n75 = To Fixed-Point(fixed-point type=w1683, number=w1692) -> (fixed-point=w1691:fxp<+/-,58,25>)
                    n76 = To Fixed-Point(fixed-point type=w1683, number=w1688) -> (fixed-point=w1687:fxp<+/-,58,25>)
                    n77 = To Fixed-Point(fixed-point type=w1683, number=w1682) -> (fixed-point=w1686:fxp<+/-,58,25>)
                    n78 = To Fixed-Point(fixed-point type=w1683, number=w1682) -> (fixed-point=w1684:fxp<+/-,58,25>)
                  }
                  frame "Data Log 9" {
                    n79 = To Fixed-Point(fixed-point type=w1701, number=w1708) -> (fixed-point=w1705:fxp<+/-,58,25>)
                    n80 = To Fixed-Point(fixed-point type=w1701, number=w1707) -> (fixed-point=w1704:fxp<+/-,58,25>)
                    n81 = To Fixed-Point(fixed-point type=w1701, number=w1706) -> (fixed-point=w1703:fxp<+/-,58,25>)
                    n82 = To Fixed-Point(fixed-point type=w1701, number=w1699) -> (fixed-point=w1702:fxp<+/-,58,25>)
                    n83 = To Fixed-Point(fixed-point type=w1701, number=w1699) -> (fixed-point=w1700:fxp<+/-,58,25>)
                  }
                  frame "Data Log 10" {
                    n84 = To Fixed-Point(fixed-point type=w1713, number=w1720) -> (fixed-point=w1719:fxp<+/-,58,25>)
                    n85 = To Fixed-Point(fixed-point type=w1713, number=w1718) -> (fixed-point=w1714:fxp<+/-,58,25>)
                    n86 = To Fixed-Point(fixed-point type=w1713, number=w1717) -> (fixed-point=w1715:fxp<+/-,58,25>)
                    n87 = To Fixed-Point(fixed-point type=w1713, number=w1711) -> (fixed-point=w1716:fxp<+/-,58,25>)
                    n88 = To Fixed-Point(fixed-point type=w1713, number=w1710) -> (fixed-point=w1712:fxp<+/-,58,25>)
                  }
                  frame "Data Log 11" {
                    n89 = To Fixed-Point(fixed-point type=w1723, number=w1733) -> (fixed-point=w1728:fxp<+/-,58,25>)
                    n90 = To Fixed-Point(fixed-point type=w1723, number=w1732) -> (fixed-point=w1727:fxp<+/-,58,25>)
                    n91 = To Fixed-Point(fixed-point type=w1723, number=w1731) -> (fixed-point=w1726:fxp<+/-,58,25>)
                    n92 = To Fixed-Point(fixed-point type=w1723, number=w1730) -> (fixed-point=w1725:fxp<+/-,58,25>)
                    n93 = To Fixed-Point(fixed-point type=w1723, number=w1722) -> (fixed-point=w1724:fxp<+/-,58,25>)
                  }
                  frame "Data Log 12" {
                    n94 = To Fixed-Point(fixed-point type=w1735, number=w1744) -> (fixed-point=w1743:fxp<+/-,58,25>)
                    n95 = To Fixed-Point(fixed-point type=w1735, number=w1739) -> (fixed-point=w1742:fxp<+/-,58,25>)
                    n96 = To Fixed-Point(fixed-point type=w1735, number=w1738) -> (fixed-point=w1741:fxp<+/-,58,25>)
                    n97 = To Fixed-Point(fixed-point type=w1735, number=w1737) -> (fixed-point=w1740:fxp<+/-,58,25>)
                    n98 = To Fixed-Point(fixed-point type=w1735, number=w1734) -> (fixed-point=w1736:fxp<+/-,58,25>)
                  }
                  frame "Data Log 13" {
                    n99 = To Fixed-Point(fixed-point type=w1746, number=w1751) -> (fixed-point=w1755:fxp<+/-,58,25>)
                    n100 = To Fixed-Point(fixed-point type=w1746, number=w1750) -> (fixed-point=w1754:fxp<+/-,58,25>)
                    n101 = To Fixed-Point(fixed-point type=w1746, number=w1749) -> (fixed-point=w1753:fxp<+/-,58,25>)
                    n102 = To Fixed-Point(fixed-point type=w1746, number=w1748) -> (fixed-point=w1752:fxp<+/-,58,25>)
                    n103 = To Fixed-Point(fixed-point type=w1746, number=w1748) -> (fixed-point=w1747:fxp<+/-,58,25>)
                  }
                  frame "Data Log 14" {
                    n104 = To Fixed-Point(fixed-point type=w1758, number=w1762) -> (fixed-point=w1766:fxp<+/-,58,25>)
                    n105 = To Fixed-Point(fixed-point type=w1758, number=w1761) -> (fixed-point=w1765:fxp<+/-,58,25>)
                    n106 = To Fixed-Point(fixed-point type=w1758, number=w1760) -> (fixed-point=w1764:fxp<+/-,58,25>)
                    n107 = To Fixed-Point(fixed-point type=w1758, number=w1757) -> (fixed-point=w1763:fxp<+/-,58,25>)
                    n108 = To Fixed-Point(fixed-point type=w1758, number=w1757) -> (fixed-point=w1759:fxp<+/-,58,25>)
                  }
                  frame "Data Log 15" {
                    n109 = To Fixed-Point(fixed-point type=w1769, number=w1773) -> (fixed-point=w1777:fxp<+/-,58,25>)
                    n110 = To Fixed-Point(fixed-point type=w1769, number=w1772) -> (fixed-point=w1776:fxp<+/-,58,25>)
                    n111 = To Fixed-Point(fixed-point type=w1769, number=w1771) -> (fixed-point=w1775:fxp<+/-,58,25>)
                    n112 = To Fixed-Point(fixed-point type=w1769, number=w1768) -> (fixed-point=w1774:fxp<+/-,58,25>)
                    n113 = To Fixed-Point(fixed-point type=w1769, number=w1768) -> (fixed-point=w1770:fxp<+/-,58,25>)
                  }
                  frame "Data Log 16" {
                    n114 = To Fixed-Point(fixed-point type=w1781, number=w1785) -> (fixed-point=w1789:fxp<+/-,58,25>)
                    n115 = To Fixed-Point(fixed-point type=w1781, number=w1784) -> (fixed-point=w1788:fxp<+/-,58,25>)
                    n116 = To Fixed-Point(fixed-point type=w1781, number=w1783) -> (fixed-point=w1787:fxp<+/-,58,25>)
                    n117 = To Fixed-Point(fixed-point type=w1781, number=w1782) -> (fixed-point=w1786:fxp<+/-,58,25>)
                    n118 = To Fixed-Point(fixed-point type=w1781, number=w1780) -> (fixed-point=w1779:fxp<+/-,58,25>)
                  }
                }
                "Number of Data Strings" <- w1578
                n119 = Build Array "Build Array"(w1592, w1591, w1590, w1580, w1572) -> (w1574:fxp<+/-,58,25>[])
              }
            }
          }
        }
        n120 = call "Loop Timer2"("Count(uSec)"="Datalog Time Period (uSec)") -> ()  [unwired: 1 out]
        n121 = for {
          N: w1555 -> [_]
          tunnel: w1548 -> [w1798] mode=indexing
          shift-right: [w1796] -> w1554
          shift-left: _ -> [w1795]
          shift-right: [w1792] -> w1549
          shift-left: _ -> [w1793]
          n122 = xnode "FIFO"("Element"=w1798, "Timeout"="Timeout FPGA FIFO1", "error in (no error)"=w1795) -> ("Timed Out?"=w1794:bool, "error out"=w1796:errorcluster)  [unwired: 1 in, 1 out]
          "FIFO Timed Out?" <- w1794
          n123 = Or(x=w1794, y=w1793) -> (x .or. y?=w1792:bool)
        }
        "FIFO Timed Out" <- w1549
        n124 = call "measure_loop_rate_FPGA.vi"() -> ("Loop Rate (Ticks)"=→"Measured Datalog Time Period (Ticks)":u32)  [unwired: 11 in]
        n125 = local read "stop case"() -> (w1550:bool)
        n126 = Unbundle By Name "Unbundle By Name"(w1554) -> ("Status?"=w1553:bool)
        n127 = Compound Arithmetic op=OR(w1553, w1549, w1550) -> (w1552:bool)
        n128 = case shown="True" w1552 {
          selector: w1552 -> [_ w1791]
          frame False {
          }
          frame True {
            n129 = local write "stop case"(w1791) -> ()
          }
        }
      }
      n130 = while {
        tunnel: [w448] -> w19
        stop <- w455 stop-if-true
        w439 = fxp<+/-,58,25> 0.0 ("fixed-point type")
        n131 = xnode "FPGA I/O Node"("FPGA I/O In"=refnum<k21> "Mod3/AI0", "FPGA I/O In"=refnum<k21> "Mod3/AI1", "FPGA I/O In"=refnum<k21> "Mod3/AI2") -> ("error out"=w448:errorcluster, "I/O Item"=w451:fxp<+/-,24,5>, "I/O Item"=w441:fxp<+/-,24,5>, "I/O Item"=w440:fxp<+/-,24,5>)  [unwired: 1 in, 3 out]
        "Mod 3 Input AI0 (V)" <- w451
        "Mod 8 Input AI1 (V)" <- w441
        "Mod 8 Input AI2 (V)" <- w440
        n132 = call "Loop Timer6"("Count(uSec)"="Analog Input Time Period (uSec)") -> ()  [unwired: 1 out]
        n133 = Multiply(x=w440, y="Mod 3 AI2 V to nm Scaling") -> (x*y=w443:fxp<+/-,64,23>)
        n134 = Multiply(x=w441, y="Mod 3 AI1 V to nm Scaling") -> (x*y=w446:fxp<+/-,64,23>)
        n135 = Multiply(x=w451, y="Mod 3 AI0 V to nm Scaling") -> (x*y=w453:fxp<+/-,64,23>)
        n136 = To Fixed-Point(fixed-point type=w439, number=w453) -> (fixed-point=→"X Stage External Reference (nm)":fxp<+/-,58,25>)
        n137 = To Fixed-Point(fixed-point type=w439, number=w446) -> (fixed-point=→"Y Stage External Reference (nm)":fxp<+/-,58,25>)
        n138 = To Fixed-Point(fixed-point type=w439, number=w443) -> (fixed-point=→"Z Stage External Reference (nm)":fxp<+/-,58,25>)
        n139 = call "measure_loop_rate_FPGA.vi"() -> ("Loop Rate (Ticks)"=→"Measured Analog Input Time Period (Ticks)":u32)  [unwired: 11 in]
        n140 = local read "stop case"() -> (w455:bool)
        n141 = case shown="True" w455 {
          frame False {
          }
          frame True {
            n142 = xnode "FPGA I/O Node"("Mod3/Stop"=TRUE ("I/O Item")) -> ()  [unwired: 1 in, 1 out]
          }
        }
      }
      n143 = while {
        shift-right: [w1805] -> _
        shift-left: u32 0 ("f") -> [w1803]
        shift-right: [w1804] -> _
        shift-left: u32 0 -> [w1802]
        stop <- w1814 stop-if-true
        n144 = case shown="\"Custom Up Down Ramp\"" "X Reference Wave Selection" {
          tunnel: "X Frequency (periods/tick)" -> [_ w1836 _ _]
          tunnel: "X Phase Offset (periods)" -> [_ w1835 _ _]
          tunnel: "X Reference Reset" -> [_ w1833 _ w1931]
          tunnel: "X White Noise Seed" -> [_ _ _ w1933]
          tunnel: "X White Noise Amplitude" -> [_ _ _ w1930]
          tunnel: "X Reference Amplitude (nm)" -> [w1821 w1828 _ w1921]
          tunnel: "X Reference DC Offset (nm)" -> [w1820 w1827 _ w1922]
          tunnel: [w1819 w1826 w1840 w1924] -> w1807
          tunnel: [_ _ w1853 _] -> w1805
          tunnel: [_ _ w1852 _] -> w1804
          tunnel: w1803 -> [_ _ w1851 _]
          tunnel: w1802 -> [_ _ w1850 _]
          tunnel: "X Ramp Period (usec)" -> [_ _ w1849 _]
          tunnel: "X Ramp Start (nm)" -> [_ _ w1838 _]
          tunnel: "X Ramp End (nm)" -> [_ _ w1839 _]
          frame "Constant", Default {
            n145 = Multiply(x=i16 1 ("y"), y=w1821) -> (x*y=w1824:fxp<+/-,56,33>)
            n146 = Add(x=w1824, y=w1820) -> (x+y=w1823:fxp<+/-,56,33>)
            n147 = To Fixed-Point(fixed-point type=fxp<+/-,58,25> 0.0, number=w1823) -> (fixed-point=w1819:fxp<+/-,58,25>)
          }
          frame "Sine Wave" {
            n148 = call "Sine Wave Generator"("frequency (periods/tick)"=w1836, "reset"=w1833, "phase offset (periods)"=w1835) -> ("sine out"=w1834:i16)  [unwired: 12 in]
            n149 = Divide(x=w1834, y=i16 32767) -> (x/y=w1829:fxp<+/-,41,18>)
            n150 = Multiply(x=w1829, y=w1828) -> (x*y=w1831:fxp<+/-,64,35>)
            n151 = Add(x=w1831, y=w1827) -> (x+y=w1830:fxp<+/-,64,36>)
            n152 = To Fixed-Point(fixed-point type=fxp<+/-,58,25> 0.0, number=w1830) -> (fixed-point=w1826:fxp<+/-,58,25>)
          }
          frame "Custom Up Down Ramp" {
            n153 = local read "Next Do Down Ramp"() -> (w1845:bool)
            n154 = Subtract(x=w1838, y=w1839) -> (x-y=w1855:fxp<+/-,17,17>)
            n155 = Less?(x=w1838, y=w1839) -> (x < y?=w1844:bool)
            n156 = Absolute Value(x=w1855) -> (abs(x)=w1854:fxp<+,16,16>)
            n157 = Not(x=w1845) -> (.not. x?=w1846:bool)
            n158 = Divide(x=w1854, y=w1849) -> (x/y=w1856:fxp<+,48,16>)
            "X Ramp Slope" <- w1856
            n159 = Compound Arithmetic op=AND(w1846, w1844) -> (w1847:bool)
            n160 = local read "X Reference Time Period (uSec)"() -> (w1848:u32)
            n161 = case shown="True" w1847 {
              tunnel: [Control_X_Up_Down_Ramp."X Down Ramp" Control_X_Up_Down_Ramp."X Up Ramp"] -> w1843
              frame False {
              }
              frame True {
              }
            }
            n162 = local read "Fly Scan Running"() -> (w1842:bool)
            n163 = case shown="True" w1842 {
              tunnel: w1843 -> [_ w1872]
              tunnel: w1848 -> [_ w1871]
              tunnel: ["X Start Marker (nm)" w1870] -> w1841
              tunnel: w1849 -> [_ w1869]
              tunnel: w1856 -> [_ w1868]
              tunnel: w1838 -> [_ w1867]
              tunnel: w1839 -> [_ w1866]
              tunnel: [_ w1865] -> w1853
              tunnel: [_ w1864] -> w1852
              tunnel: w1851 -> [_ w1863]
              tunnel: w1850 -> [_ w1862]
              frame False {
                n164 = local write "Next Do Down Ramp"(FALSE ("Restart Up Ramp")) -> ()
                n165 = local write "Y Ramp Drop"(FALSE ("Y Toggle 1")) -> ()
              }
              frame True {
                n166 = case shown="\"X Down Ramp\"" w1872 {
                  tunnel: [w1891 _] -> w1865
                  tunnel: w1863 -> [w1890 _]
                  tunnel: w1871 -> [w1887 w1912]
                  tunnel: w1869 -> [w1886 w1908]
                  tunnel: w1867 -> [w1877 w1899]
                  tunnel: w1866 -> [w1875 w1900]
                  tunnel: [_ w1915] -> w1864
                  tunnel: w1862 -> [_ w1914]
                  tunnel: w1868 -> [w1882 w1906]
                  tunnel: [w1879 w1902] -> w1870
                  frame "X Up Ramp", Default {
                    n167 = Increment(x=w1890) -> (x+1=w1888:u32)
                    n168 = Multiply(x=w1888, y=w1887) -> (x*y=w1883:u32)
                    n169 = Multiply(x=w1883, y=w1882) -> (x*y=w1881:fxp<+,64,48>)
                    n170 = Less Or Equal?(x=w1883, y=w1886) -> (x <= y?=w1885:bool)
                    "X Ramp Mid Range" <- w1885
                    n171 = Add(x=w1881, y=w1877) -> (x+y=w1880:fxp<+/-,64,50>)
                    n172 = Greater?(x=w1883, y=w1886) -> (0:w1876:bool)
                    "If True End X Up Ramp" <- w1876
                    n173 = local write "Y Ramp Drop"(FALSE ("Y Ramp Drop")) -> ()
                    n174 = case shown="True" w1876 {
                      frame False {
                      }
                      frame True {
                        n175 = local write "Start or middle"(TRUE ("Start or middle")) -> ()
                        n176 = local write "Fly Scan Start"(FALSE ("Fly Scan Start")) -> ()
                        "Y Ramp Drop" <- TRUE ("Boolean")
                        "Next Do Down Ramp" <- TRUE
                      }
                    }
                    n177 = Greater?(x=w1880, y=w1875) -> (0:w1878:bool)
                    n178 = Select(t=w1888, s=w1885, f=u32 0) -> (s? t:f=w1889:u32)
                    n179 = Select(t=w1875, s=w1878, f=w1880) -> (s? t:f=w1879:fxp<+/-,64,50>)
                    n180 = Select(t=u32 0, s=w1876, f=w1889) -> (s? t:f=w1891:u32)
                    "Continue Run" <- TRUE ("Fly Scan Running")
                  }
                  frame "X Down Ramp" {
                    n181 = Increment(x=w1914) -> (x+1=w1913:u32)
                    n182 = Multiply(x=w1913, y=w1912) -> (x*y=w1907:u32)
                    n183 = Multiply(x=w1907, y=w1906) -> (x*y=w1905:fxp<+,64,48>)
                    n184 = Less Or Equal?(x=w1907, y=w1908) -> (x <= y?=w1911:bool)
                    n185 = Greater?(x=w1907, y=w1908) -> (0:w1901:bool)
                    "If True End X Down Ramp" <- w1901
                    n186 = local write "Y Ramp Drop"(FALSE ("Y Ramp Drop")) -> ()
                    n187 = Subtract(x=w1900, y=w1905) -> (x-y=w1903:fxp<+/-,64,50>)
                    n188 = case shown="True" w1901 {
                      frame False {
                      }
                      frame True {
                        n189 = local write "Y Ramp Drop"(TRUE ("Start Scan")) -> ()
                        n190 = local write "Fly Scan Start"(FALSE ("Fly Scan Start")) -> ()
                        n191 = local write "Start or middle"(TRUE ("Start or middle")) -> ()
                        n192 = local write "Next Do Down Ramp"(FALSE ("Next Do Down Ramp")) -> ()
                      }
                    }
                    n193 = Less?(x=w1903, y=w1899) -> (x < y?=w1904:bool)
                    n194 = Select(t=w1913, s=w1911, f=u32 0) -> (s? t:f=w1909:u32)
                    n195 = local write "Continue Run"(TRUE ("Fly Scan Running")) -> ()
                    n196 = Select(t=w1899, s=w1904, f=w1903) -> (s? t:f=w1902:fxp<+/-,64,50>)
                    n197 = Select(t=u32 0, s=w1901, f=w1909) -> (s? t:f=w1915:u32)
                  }
                }
              }
            }
            n198 = To Fixed-Point(fixed-point type=fxp<+/-,58,25> 0.0, number=w1841) -> (fixed-point=w1840:fxp<+/-,58,25>)
          }
          frame "Filtered White Noise" {
            n199 = call "White Noise Generator"("seed"=w1933, "reset"=w1931, "amplitude"=w1930) -> ("white noise out"=w1932:i16)  [unwired: 12 in]
            n200 = xnode "Butterworth Filter"("input data"=w1932, "reset"=w1931) -> ("output data"=w1928:i16)  [unwired: 1 in]
            n201 = Divide(x=w1928, y=i16 32767) -> (x/y=w1923:fxp<+/-,41,18>)
            n202 = Multiply(x=w1923, y=w1921) -> (x*y=w1926:fxp<+/-,64,35>)
            n203 = Add(x=w1926, y=w1922) -> (x+y=w1925:fxp<+/-,64,36>)
            n204 = To Fixed-Point(fixed-point type=fxp<+/-,58,25> 0.0, number=w1925) -> (fixed-point=w1924:fxp<+/-,58,25>)
          }
        }
        "X Stage Reference (nm)" <- w1807
        n205 = call "measure_loop_rate_FPGA.vi"() -> ("Loop Rate (Ticks)"=→"Measured X Reference Time Period (Ticks)":u32)  [unwired: 11 in]
        n206 = local read "stop case"() -> (w1814:bool)
        n207 = call "Loop Timer"("Count(uSec)"="X Reference Time Period (uSec)") -> ()  [unwired: 1 out]
      }
      n208 = while {
        shift-right: [w304] -> _
        shift-left: i16 0 -> [w303]
        shift-right: [w302] -> _
        shift-left: i16 0 -> [w301]
        stop <- w314 stop-if-true
        n209 = local read "Fly Scan Running"() -> (w293:bool)
        n210 = case shown="\"Custom Square Wave \", Default" "Trigger Wave Generator" {
          tunnel: [w330 w374 w396] -> w305
          tunnel: [w328 _ _] -> w304
          tunnel: w303 -> [w327 _ _]
          tunnel: [w321 _ _] -> w302
          tunnel: w301 -> [w320 _ _]
          tunnel: "DT Reset" -> [_ w380 w401]
          tunnel: "DT Frequency (periods/tick)" -> [_ w379 w400]
          tunnel: "DT Phase Offset (periods)" -> [_ w378 w399]
          tunnel: "DT Duty Cycle (periods)" -> [_ w377 _]
          tunnel: "DT Reference Amplitude (V)" -> [_ w376 w398]
          tunnel: "DT Reference DC Offset (V)" -> [_ w375 w397]
          tunnel: w293 -> [w315 w373 w395]
          frame "Custom Square Wave ", Default {
            n211 = local read "If True End Trigger High"() -> (w319:bool)
            n212 = local read "If True End Trigger Low"() -> (w318:bool)
            n213 = Not(x=w319) -> (.not. x?=w317:bool)
            n214 = Compound Arithmetic op=AND(w318, w317) -> (w316:bool)
            n215 = local read "Trigger Generation Time Period (uSec)"() -> (w326:u32)
            n216 = case shown="True" w316 {
              tunnel: [Detector_Trigger_Control."Trigger Low" Detector_Trigger_Control."Trigger High"] -> w329
              frame False {
              }
              frame True {
              }
            }
            n217 = case shown="True" w315 {
              tunnel: [fxp<+/-,20,5> 0.0 ("Trigger High Level (V)") w336] -> w330
              tunnel: w329 -> [_ w344]
              tunnel: [_ w343] -> w328
              tunnel: w327 -> [_ w342]
              tunnel: w326 -> [_ w341]
              tunnel: "Trigger High Period (usec)" -> [_ w340]
              tunnel: "Trigger Low Period (usec)" -> [_ w339]
              tunnel: "Trigger High Level (V)" -> [_ w338]
              tunnel: "Trigger Low Level (V)" -> [_ w337]
              tunnel: [_ w335] -> w321
              tunnel: w320 -> [_ w334]
              frame False {
                n218 = local write "If True End Trigger High"(FALSE ("If True End Trigger High")) -> ()
                n219 = local write "If True End Trigger Low"(TRUE ("If True End Trigger Low")) -> ()
              }
              frame True {
                n220 = case shown="\"Trigger High\", Default" w344 {
                  tunnel: [w355 _] -> w343
                  tunnel: w342 -> [w354 _]
                  tunnel: w341 -> [w351 w365]
                  tunnel: w340 -> [w349 _]
                  tunnel: w339 -> [_ w363]
                  tunnel: w338 -> [w346 _]
                  tunnel: w337 -> [_ w358]
                  tunnel: [w346 w358] -> w336
                  tunnel: [_ w368] -> w335
                  tunnel: w334 -> [_ w367]
                  frame "Trigger High", Default {
                    n221 = Increment(x=w354) -> (x+1=w352:i16)
                    n222 = Multiply(x=w352, y=w351) -> (x*y=w350:u32)
                    n223 = Less Or Equal?(x=w350, y=w349) -> (x <= y?=w348:bool)
                    "Trigger Mid High" <- w348
                    n224 = Greater?(x=w350, y=w349) -> (0:w345:bool)
                    "If True End Trigger High" <- w345
                    n225 = case shown="True" w345 {
                      frame False {
                      }
                      frame True {
                        n226 = local write "If True End Trigger Low"(FALSE) -> ()
                      }
                    }
                    n227 = Select(t=w352, s=w348, f=i16 0) -> (s? t:f=w353:i16)
                    n228 = Select(t=i16 0, s=w345, f=w353) -> (s? t:f=w355:i16)
                  }
                  frame "Trigger Low" {
                    n229 = Increment(x=w367) -> (x+1=w366:i16)
                    n230 = Multiply(x=w366, y=w365) -> (x*y=w364:u32)
                    n231 = Less Or Equal?(x=w364, y=w363) -> (x <= y?=w362:bool)
                    n232 = Greater?(x=w364, y=w363) -> (0:w359:bool)
                    "If True End Trigger Low" <- w359
                    n233 = case shown="True" w359 {
                      frame False {
                      }
                      frame True {
                        n234 = local write "If True End Trigger High"(FALSE) -> ()
                      }
                    }
                    n235 = Select(t=w366, s=w362, f=i16 0) -> (s? t:f=w360:i16)
                    n236 = Select(t=i16 0, s=w359, f=w360) -> (s? t:f=w368:i16)
                  }
                }
              }
            }
          }
          frame "Square Wave 1" {
            n237 = case shown="True" w373 {
              tunnel: w380 -> [_ w388]
              tunnel: w379 -> [_ w387]
              tunnel: w378 -> [_ w386]
              tunnel: w377 -> [_ w385]
              tunnel: w376 -> [_ w384]
              tunnel: w375 -> [_ w383]
              tunnel: [fxp<+/-,58,25> 0.0 ("fixed-point type") w382] -> w374
              frame False {
              }
              frame True {
                n238 = call "Square Wave Generator"("frequency (periods/tick)"=w387, "reset"=w388, "phase offset (periods)"=w386, "duty cycle (periods)"=w385) -> ("square wave out"=w394:i16)  [unwired: 11 in]
                n239 = Divide(x=w394, y=i16 32767) -> (x/y=w392:fxp<+/-,41,18>)
                n240 = Multiply(x=w392, y=w384) -> (x*y=w391:fxp<+/-,64,35>)
                n241 = Add(x=w391, y=w383) -> (x+y=w390:fxp<+/-,64,36>)
                n242 = To Fixed-Point(fixed-point type=fxp<+/-,58,25> 0.0, number=w390) -> (fixed-point=w382:fxp<+/-,58,25>)
              }
            }
          }
          frame "Square Wave 2" {
            n243 = case shown="True" w395 {
              tunnel: w400 -> [_ w408]
              tunnel: w399 -> [_ w407]
              tunnel: w401 -> [_ w406]
              tunnel: w398 -> [_ w405]
              tunnel: w397 -> [_ w404]
              tunnel: [fxp<+/-,58,25> 0.0 ("fixed-point type") w403] -> w396
              frame False {
              }
              frame True {
                w414 = fxp<+/-,32,16> 0.0 ("fixed-point type")
                n244 = call "Sine Wave Generator3"("frequency (periods/tick)"=w408, "reset"=w406, "phase offset (periods)"=w407) -> ("sine out"=w413:i16)  [unwired: 12 in]
                n245 = Divide(x=w413, y=i16 32767) -> (x/y=w434:fxp<+/-,41,18>)
                n246 = Greater?(x=w434, y=w414) -> (0:w421:bool)
                n247 = Equal?(x=w434, y=w414) -> (x = y?=w422:bool)
                n248 = Less?(x=w434, y=w414) -> (x < y?=w420:bool)
                n249 = Not(x=w421) -> (.not. x?=w418:bool)
                n250 = Not(x=w422) -> (.not. x?=w417:bool)
                n251 = Not(x=w420) -> (.not. x?=w419:bool)
                n252 = Compound Arithmetic op=AND(w421, w417, w419) -> (w423:bool)
                n253 = Compound Arithmetic op=AND(w418, w422, w419) -> (w416:bool)
                n254 = Compound Arithmetic op=AND(w418, w417, w420) -> (w415:bool)
                n255 = Select(t=fxp<+/-,2,2> 1.0 ("fixed-point type"), s=w423, f=fxp<+/-,2,2> 0.0 ("fixed-point type")) -> (s? t:f=w427:fxp<+/-,2,2>)
                n256 = Select(t=fxp<+/-,2,2> 0.0 ("fixed-point type"), s=w416, f=fxp<+/-,2,2> 0.0 ("fixed-point type")) -> (s? t:f=w426:fxp<+/-,2,2>)
                n257 = Select(t=fxp<+/-,2,2> -1.0 ("fixed-point type"), s=w415, f=fxp<+/-,2,2> 0.0 ("fixed-point type")) -> (s? t:f=w424:fxp<+/-,2,2>)
                n258 = Add(x=w427, y=w426) -> (x+y=w425:fxp<+/-,3,3>)
                n259 = Add(x=w425, y=w424) -> (x+y=w410:fxp<+/-,4,4>)
                n260 = Multiply(x=w410, y=w405) -> (x*y=w411:fxp<+/-,43,20>)
                n261 = Add(x=w411, y=w404) -> (x+y=w409:fxp<+/-,43,20>)
                n262 = To Fixed-Point(fixed-point type=fxp<+/-,58,25> 0.0, number=w409) -> (fixed-point=w403:fxp<+/-,58,25>)
              }
            }
          }
        }
        n263 = call "measure_loop_rate_FPGA.vi"() -> ("Loop Rate (Ticks)"=→"Measured Trigger Gen Time Period (Ticks)":u32)  [unwired: 11 in]
        n264 = To Fixed-Point(fixed-point type=fxp<+/-,20,5> 0.0, number=w305) -> (fixed-point=w306:fxp<+/-,20,5>)
        n265 = In Range and Coerce(upper limit="Detector Trigger Upper Limit (V)", x=w306, lower limit="Detector Trigger Lower Limit (V)") -> (coerced(x)=→"Detector Trigger (V)":fxp<+/-,20,5>, In Range?=→"Detector Trigger In Range?":bool)
        n266 = call "Loop Timer7"("Count(uSec)"="Trigger Generation Time Period (uSec)") -> ()  [unwired: 1 out]
        n267 = local read "stop case"() -> (w314:bool)
      }
      n268 = while {
        stop <- w43 stop-if-true
        n269 = case shown="\"Filtered White Noise\"" "Z Reference Wave Selection" {
          tunnel: "Z Reference Reset" -> [_ w73 w80 w96 w129]
          tunnel: "Z Frequency (periods/tick)" -> [_ w72 w79 w95 _]
          tunnel: "Z Phase Offset (periods)" -> [_ w71 w78 w94 _]
          tunnel: "Z White Noise Seed" -> [_ _ _ _ w131]
          tunnel: "Z White Noise Amplitude" -> [_ _ _ _ w130]
          tunnel: "Z Reference DC Offset (nm)" -> [w55 w64 w75 w86 w120]
          tunnel: "Z Reference Amplitude (nm)" -> [w56 w65 w74 w88 w121]
          tunnel: [w57 w62 w76 w91 w119] -> w44
          frame "Constant", Default {
            n270 = Multiply(x=i16 1 ("y"), y=w56) -> (x*y=w60:fxp<+/-,56,33>)
            n271 = Add(x=w60, y=w55) -> (x+y=w59:fxp<+/-,56,33>)
            n272 = To Fixed-Point(fixed-point type=fxp<+/-,58,25> 0.0, number=w59) -> (fixed-point=w57:fxp<+/-,58,25>)
          }
          frame "Sine Wave" {
            n273 = call "Sine Wave Generator2"("frequency (periods/tick)"=w72, "reset"=w73, "phase offset (periods)"=w71) -> ("sine out"=w66:i16)  [unwired: 12 in]
            n274 = Divide(x=w66, y=i16 32767) -> (x/y=w69:fxp<+/-,41,18>)
            n275 = Multiply(x=w69, y=w65) -> (x*y=w68:fxp<+/-,64,35>)
            n276 = Add(x=w68, y=w64) -> (x+y=w67:fxp<+/-,64,36>)
            n277 = To Fixed-Point(fixed-point type=fxp<+/-,58,25> 0.0, number=w67) -> (fixed-point=w62:fxp<+/-,58,25>)
          }
          frame "Sawtooth Wave" {
            n278 = call "Saw Wave Generator.vi"("frequency (periods/tick)"=w79, "reset"=w80, "phase offset (periods)"=w78) -> ("saw out"=w77:i16)  [unwired: 12 in]
            n279 = Divide(x=w77, y=i16 32767) -> (x/y=w84:fxp<+/-,41,18>)
            n280 = Multiply(x=w84, y=w74) -> (x*y=w83:fxp<+/-,64,35>)
            n281 = Add(x=w83, y=w75) -> (x+y=w82:fxp<+/-,64,36>)
            n282 = To Fixed-Point(fixed-point type=fxp<+/-,58,25> 0.0, number=w82) -> (fixed-point=w76:fxp<+/-,58,25>)
          }
          frame "Square Wave" {
            w97 = fxp<+/-,32,16> 0.0 ("fixed-point type")
            n283 = call "Sine Wave Generator5"("frequency (periods/tick)"=w95, "reset"=w96, "phase offset (periods)"=w94) -> ("sine out"=w93:i16)  [unwired: 12 in]
            n284 = Divide(x=w93, y=i16 32767) -> (x/y=w117:fxp<+/-,41,18>)
            n285 = Greater?(x=w117, y=w97) -> (0:w104:bool)
            n286 = Equal?(x=w117, y=w97) -> (x = y?=w105:bool)
            n287 = Less?(x=w117, y=w97) -> (x < y?=w103:bool)
            n288 = Not(x=w104) -> (.not. x?=w101:bool)
            n289 = Not(x=w105) -> (.not. x?=w100:bool)
            n290 = Not(x=w103) -> (.not. x?=w102:bool)
            n291 = Compound Arithmetic op=AND(w104, w100, w102) -> (w106:bool)
            n292 = Compound Arithmetic op=AND(w101, w105, w102) -> (w99:bool)
            n293 = Compound Arithmetic op=AND(w101, w100, w103) -> (w98:bool)
            n294 = Select(t=fxp<+/-,2,2> 1.0 ("fixed-point type"), s=w106, f=fxp<+/-,2,2> 0.0 ("fixed-point type")) -> (s? t:f=w110:fxp<+/-,2,2>)
            n295 = Select(t=fxp<+/-,2,2> 0.0 ("fixed-point type"), s=w99, f=fxp<+/-,2,2> 0.0 ("fixed-point type")) -> (s? t:f=w109:fxp<+/-,2,2>)
            n296 = Select(t=fxp<+/-,2,2> -1.0 ("fixed-point type"), s=w98, f=fxp<+/-,2,2> 0.0 ("fixed-point type")) -> (s? t:f=w107:fxp<+/-,2,2>)
            n297 = Add(x=w110, y=w109) -> (x+y=w108:fxp<+/-,3,3>)
            n298 = Add(x=w108, y=w107) -> (x+y=w89:fxp<+/-,4,4>)
            n299 = Multiply(x=w89, y=w88) -> (x*y=w90:fxp<+/-,43,20>)
            n300 = Add(x=w90, y=w86) -> (x+y=w87:fxp<+/-,43,20>)
            n301 = To Fixed-Point(fixed-point type=fxp<+/-,58,25> 0.0, number=w87) -> (fixed-point=w91:fxp<+/-,58,25>)
          }
          frame "Filtered White Noise" {
            n302 = call "White Noise Generator3"("seed"=w131, "reset"=w129, "amplitude"=w130) -> ("white noise out"=w128:i16)  [unwired: 12 in]
            n303 = xnode "Butterworth Filter"("input data"=w128, "reset"=w129) -> ("output data"=w123:i16)  [unwired: 1 in]
            n304 = Divide(x=w123, y=i16 32767) -> (x/y=w126:fxp<+/-,41,18>)
            n305 = Multiply(x=w126, y=w121) -> (x*y=w125:fxp<+/-,64,35>)
            n306 = Add(x=w125, y=w120) -> (x+y=w124:fxp<+/-,64,36>)
            n307 = To Fixed-Point(fixed-point type=fxp<+/-,58,25> 0.0, number=w124) -> (fixed-point=w119:fxp<+/-,58,25>)
          }
        }
        "Z Stage Reference (nm)" <- w44
        n308 = call "measure_loop_rate_FPGA.vi"() -> ("Loop Rate (Ticks)"=→"Measured Z Reference Time Period (Ticks)":u32)  [unwired: 11 in]
        n309 = local read "stop case"() -> (w43:bool)
        n310 = call "Loop Timer10"("Count(uSec)"="Z Reference Time Period (uSec)") -> ()  [unwired: 1 out]
      }
      n311 = while {
        shift-right: [w148] -> _
        shift-left: _ -> [w143]
        shift-right: [w147] -> _
        shift-left: u32 0 ("f") -> [w145]
        shift-right: [w146] -> _
        shift-left: u32 0 -> [w144]
        stop <- w149 stop-if-true
        n312 = case shown="\"Custom Ramp Wave\"" "Y Reference Wave Selection" {
          tunnel: "Y Reference Amplitude (nm)" -> [w166 w170 _ w270]
          tunnel: "Y Reference DC Offset (nm)" -> [w165 w169 _ w269]
          tunnel: [w161 w168 w196 w266] -> w157
          tunnel: "Y Frequency (periods/tick)" -> [_ w179 _ _]
          tunnel: "Y Phase Offset (periods)" -> [_ w178 _ _]
          tunnel: "Y Reference Reset" -> [_ w177 _ w275]
          tunnel: "Y White Noise Seed" -> [_ _ _ w278]
          tunnel: "Y White Noise Amplitude" -> [_ _ _ w277]
          tunnel: [_ _ w194 _] -> w148
          tunnel: [_ _ w191 _] -> w147
          tunnel: [_ _ w190 _] -> w146
          tunnel: w145 -> [_ _ w189 _]
          tunnel: w144 -> [_ _ w188 _]
          tunnel: w143 -> [_ _ w186 _]
          tunnel: "Y Ramp Period (usec)" -> [_ _ w182 _]
          tunnel: "Y Ramp End (nm)" -> [_ _ w181 _]
          tunnel: "Y Ramp Start (nm)" -> [_ _ w180 _]
          frame "Constant", Default {
            n313 = Multiply(x=i16 1 ("y"), y=w166) -> (x*y=w164:fxp<+/-,56,33>)
            n314 = Add(x=w164, y=w165) -> (x+y=w163:fxp<+/-,56,33>)
            n315 = To Fixed-Point(fixed-point type=fxp<+/-,58,25> 0.0, number=w163) -> (fixed-point=w161:fxp<+/-,58,25>)
          }
          frame "Sine Wave" {
            n316 = call "Sine Wave Generator4"("frequency (periods/tick)"=w179, "reset"=w177, "phase offset (periods)"=w178) -> ("sine out"=w176:i16)  [unwired: 12 in]
            n317 = Divide(x=w176, y=i16 32767) -> (x/y=w174:fxp<+/-,41,18>)
            n318 = Multiply(x=w174, y=w170) -> (x*y=w173:fxp<+/-,64,35>)
            n319 = Add(x=w173, y=w169) -> (x+y=w172:fxp<+/-,64,36>)
            n320 = To Fixed-Point(fixed-point type=fxp<+/-,58,25> 0.0, number=w172) -> (fixed-point=w168:fxp<+/-,58,25>)
          }
          frame "Custom Ramp Wave" {
            n321 = Subtract(x=w180, y=w181) -> (x-y=w201:fxp<+/-,17,17>)
            n322 = Less?(x=w180, y=w181) -> (x < y?=w185:bool)
            n323 = Absolute Value(x=w201) -> (abs(x)=w200:fxp<+,16,16>)
            n324 = local read "Continue Run"() -> (w184:bool)
            n325 = Divide(x=w200, y=w182) -> (x/y=w202:fxp<+,48,16>)
            "Y Ramp Slope" <- w202
            n326 = local read "Start or middle"() -> (w198:bool)
            n327 = local read "Y Reference Time Period (uSec)"() -> (w187:u32)
            n328 = case shown="True" w185 {
              tunnel: [Control_Y_Up_Down_Ramp."Y Down Ramp" Control_Y_Up_Down_Ramp."Y Up Ramp"] -> w183
              frame False {
              }
              frame True {
              }
            }
            n329 = Compound Arithmetic op=OR("Fly Scan Start", w184) -> (w193:bool)
            "Fly Scan Running" <- w193
            n330 = Select(t=w186, s=w198, f=w180) -> (s? t:f=w199:fxp<+/-,58,25>)
            n331 = case shown="True" w193 {
              tunnel: w183 -> [_ w219]
              tunnel: w187 -> [_ w218]
              tunnel: ["Y Start Marker (nm)" w217] -> w197
              tunnel: w182 -> [_ w216]
              tunnel: w202 -> [_ w215]
              tunnel: w180 -> [_ w214]
              tunnel: w181 -> [_ w213]
              tunnel: [_ w212] -> w191
              tunnel: [_ w211] -> w190
              tunnel: w189 -> [_ w210]
              tunnel: w188 -> [_ w209]
              tunnel: [_ w208] -> w194
              tunnel: w199 -> [_ w207]
              frame False {
                "Start or middle" <- FALSE ("Start or middle")
              }
              frame True {
                n332 = case shown="\"Y Down Ramp\"" w219 {
                  tunnel: [w238 _] -> w212
                  tunnel: w210 -> [w237 _]
                  tunnel: w218 -> [w234 w255]
                  tunnel: w216 -> [w233 w251]
                  tunnel: w214 -> [w223 _]
                  tunnel: w213 -> [w227 w244]
                  tunnel: [_ w258] -> w211
                  tunnel: w209 -> [_ w257]
                  tunnel: w215 -> [w229 _]
                  tunnel: [w221 w240] -> w217
                  tunnel: [_ w240] -> w208
                  tunnel: w207 -> [_ w242]
                  frame "Y Up Ramp", Default {
                    n333 = Increment(x=w237) -> (x+1=w235:u32)
                    n334 = Multiply(x=w235, y=w234) -> (x*y=w230:u32)
                    n335 = Multiply(x=w230, y=w229) -> (x*y=w228:fxp<+,64,48>)
                    n336 = Less Or Equal?(x=w230, y=w233) -> (x <= y?=w232:bool)
                    "Ramp Mid Range" <- w232
                    n337 = Add(x=w228, y=w223) -> (x+y=w226:fxp<+/-,64,50>)
                    n338 = Greater?(x=w230, y=w233) -> (0:w222:bool)
                    "If True End Up Ramp" <- w222
                    n339 = Greater?(x=w226, y=w227) -> (0:w224:bool)
                    n340 = Select(t=w235, s=w232, f=i16 0) -> (s? t:f=w236:u32)
                    n341 = Select(t=w223, s=w224, f=w226) -> (s? t:f=w225:fxp<+/-,64,50>)
                    n342 = Select(t=i16 0, s=w222, f=w236) -> (s? t:f=w238:u32)
                    n343 = To Fixed-Point(fixed-point type=fxp<+/-,58,25> 0.0, number=w225) -> (fixed-point=w221:fxp<+/-,58,25>)
                  }
                  frame "Y Down Ramp" {
                    n344 = Increment(x=w257) -> (x+1=w256:u32)
                    n345 = local read "Y Ramp Drop"() -> (w248:bool)
                    n346 = Multiply(x=w256, y=w255) -> (x*y=w250:u32)
                    n347 = Less Or Equal?(x=w250, y=w251) -> (x <= y?=w254:bool)
                    n348 = Greater?(x=w250, y=w251) -> (0:w249:bool)
                    "If True End Y Down Ramp" <- w249
                    n349 = case shown="True" w248 {
                      tunnel: "Y Ramp Drop Size (nm)" -> [_ w263]
                      tunnel: [w260 w262] -> w246
                      tunnel: w242 -> [w260 w261]
                      frame False {
                      }
                      frame True {
                        n350 = Subtract(x=w261, y=w263) -> (x-y=w262:fxp<+/-,59,26>)
                      }
                    }
                    n351 = Select(t=w256, s=w254, f=u32 0) -> (s? t:f=w252:u32)
                    n352 = To Fixed-Point(fixed-point type=fxp<+/-,58,25> 0.0, number=w246) -> (fixed-point=w241:fxp<+/-,58,25>)
                    n353 = Less?(x=w241, y=w244) -> (x < y?=w243:bool)
                    n354 = case shown="True" w243 {
                      frame False {
                      }
                      frame True {
                        n355 = local write "Fly Scan Running"(FALSE ("Fly Scan Running")) -> ()
                        n356 = local write "Continue Run"(FALSE ("Start Scan")) -> ()
                      }
                    }
                    n357 = Select(t=u32 0, s=w249, f=w252) -> (s? t:f=w258:u32)
                    n358 = Select(t=w242, s=w243, f=w241) -> (s? t:f=w240:fxp<+/-,58,25>)
                  }
                }
              }
            }
            n359 = To Fixed-Point(fixed-point type=fxp<+/-,58,25> 0.0, number=w197) -> (fixed-point=w196:fxp<+/-,58,25>)
          }
          frame "Filtered White Noise" {
            n360 = call "White Noise Generator2"("seed"=w278, "reset"=w275, "amplitude"=w277) -> ("white noise out"=w276:i16)  [unwired: 12 in]
            n361 = xnode "Butterworth Filter"("input data"=w276, "reset"=w275) -> ("output data"=w273:i16)  [unwired: 1 in]
            n362 = Divide(x=w273, y=i16 32767) -> (x/y=w272:fxp<+/-,41,18>)
            n363 = Multiply(x=w272, y=w270) -> (x*y=w271:fxp<+/-,64,35>)
            n364 = Add(x=w271, y=w269) -> (x+y=w268:fxp<+/-,64,36>)
            n365 = To Fixed-Point(fixed-point type=fxp<+/-,58,25> 0.0, number=w268) -> (fixed-point=w266:fxp<+/-,58,25>)
          }
        }
        "Y Stage Reference (nm)" <- w157
        n366 = call "measure_loop_rate_FPGA.vi"() -> ("Loop Rate (Ticks)"=→"Measured Y Reference Time Period (Ticks)":u32)  [unwired: 11 in]
        n367 = local read "stop case"() -> (w149:bool)
        n368 = call "Loop Timer9"("Count(uSec)"="Y Reference Time Period (uSec)") -> ()  [unwired: 1 out]
      }
      n369 = while {
        stop <- w484 stop-if-true
        w463 = fxp<+/-,58,25> 0.0 ("fixed-point type")
        n370 = local read "32 bit Count Sample  Y"() -> (w460:i32)
        n371 = local read "32 bit Count Sample  Z"() -> (w457:i32)
        n372 = local read "32 bit Count Sample X"() -> (w461:i32)
        n373 = local read "32 bit Count Optics  Y"() -> (w477:i32)
        n374 = local read "32 bit Count Optics  Z"() -> (w473:i32)
        n375 = local read "32 bit Count Optics X"() -> (w483:i32)
        n376 = Multiply(x=w483, y="Optics X Stage Resolution (nm)") -> (x*y=w480:fxp<+/-,64,35>)
        "Optics X Stage Displacement raw (nm)" <- w480
        n377 = Multiply(x=w461, y="Sample X Stage Resolution (nm)") -> (x*y=w469:fxp<+/-,64,35>)
        "Sample X Stage Displacement raw (nm)" <- w469
        n378 = Multiply(x=w477, y="Optics Y Stage Resolution (nm)") -> (x*y=w475:fxp<+/-,64,35>)
        "Optics Y Stage Displacement raw (nm)" <- w475
        n379 = Multiply(x=w460, y="Sample Y Stage Resolution (nm)") -> (x*y=w467:fxp<+/-,64,35>)
        "Sample Y Stage Displacement raw (nm)" <- w467
        n380 = Multiply(x=w473, y="Optics Z Stage Resolution (nm)") -> (x*y=w471:fxp<+/-,64,35>)
        "Optics Z Stage Displacement raw (nm)" <- w471
        n381 = Multiply(x=w457, y="Sample Z Stage Resolution (nm)") -> (x*y=w465:fxp<+/-,64,35>)
        "Sample Z Stage Displacement raw (nm)" <- w465
        n382 = call "Loop Timer5"("Count(uSec)"="Plant Output Time Period (uSec)") -> ()  [unwired: 1 out]
        n383 = call "measure_loop_rate_FPGA.vi"() -> ("Loop Rate (Ticks)"=→"Measured Plant Output Time Period (Ticks)":u32)  [unwired: 11 in]
        n384 = To Fixed-Point(fixed-point type=w463, number=w480) -> (fixed-point=→"Optics X Stage Displacement (nm)":fxp<+/-,58,25>)
        n385 = To Fixed-Point(fixed-point type=w463, number=w475) -> (fixed-point=→"Optics Y Stage Displacement (nm)":fxp<+/-,58,25>)
        n386 = To Fixed-Point(fixed-point type=w463, number=w471) -> (fixed-point=→"Optics Z Stage Displacement (nm)":fxp<+/-,58,25>)
        n387 = To Fixed-Point(fixed-point type=w463, number=w469) -> (fixed-point=→"Sample X Stage Displacement (nm)":fxp<+/-,58,25>)
        n388 = To Fixed-Point(fixed-point type=w463, number=w467) -> (fixed-point=→"Sample Y Stage Displacement (nm)":fxp<+/-,58,25>)
        n389 = To Fixed-Point(fixed-point type=w463, number=w465) -> (fixed-point=→"Sample Z Stage Displacement (nm)":fxp<+/-,58,25>)
        n390 = local read "stop case"() -> (w484:bool)
      }
      n391 = while {
        tunnel: [w609] -> w20
        stop <- w612 stop-if-true
        n392 = local read "PI X-Stage Input (V)"() -> (w608:fxp<+/-,20,5>)
        n393 = local read "PI Y-Stage Input (V)"() -> (w607:fxp<+/-,20,5>)
        n394 = local read "PI Z-Stage Input (V)"() -> (w606:fxp<+/-,20,5>)
        n395 = xnode "FPGA I/O Node"("I/O Item"=w608, "FPGA I/O In"=refnum<k21> "Mod8/AO0", "I/O Item"=w607, "FPGA I/O In"=refnum<k21> "Mod8/AO1") -> ("error out"=w605:errorcluster)  [unwired: 1 in, 2 out]
        n396 = xnode "FPGA I/O Node"("I/O Item"=w606, "FPGA I/O In"=refnum<k21> "Mod8/AO2") -> ("error out"=w610:errorcluster)  [unwired: 1 in, 1 out]
        n397 = call "Loop Timer4"("Count(uSec)"="Controller Output Time Period (uSec)") -> ()  [unwired: 1 out]
        n398 = Merge Errors "Merge Errors"(w605, w610) -> (w609:errorcluster)
        n399 = call "measure_loop_rate_FPGA.vi"() -> ("Loop Rate (Ticks)"=→"Measured Controller Output Time Period (Ticks)":u32)  [unwired: 11 in]
        n400 = local read "stop case"() -> (w612:bool)
      }
      n401 = node-c288(refnum<k21> "40 MHz Onboard Clock" ("Source Name"), w21) -> (w29:T10)
      n402 = while {
        shift-right: [w686] -> _
        shift-left: _ -> [w677]
        shift-right: [w685] -> _
        shift-left: _ -> [w676]
        shift-right: [w684] -> _
        shift-left: _ -> [w675]
        shift-right: [w683] -> _
        shift-left: _ -> [w674]
        shift-right: [w682] -> _
        shift-left: _ -> [w673]
        shift-right: [w681] -> _
        shift-left: _ -> [w672]
        shift-right: [w680] -> _
        shift-left: _ -> [w671]
        shift-right: [w679] -> _
        shift-left: _ -> [w670]
        shift-right: [w678] -> _
        shift-left: _ -> [w669]
        shift-right: [w663] -> _
        shift-left: _ -> [w662]
        shift-right: [w661] -> _
        shift-left: _ -> [w660]
        shift-right: [w659] -> _
        shift-left: _ -> [w658]
        shift-right: [w657] -> _
        shift-left: _ -> [w656]
        shift-right: [w655] -> _
        shift-left: _ -> [w654]
        shift-right: [w653] -> _
        shift-left: _ -> [w652]
        shift-right: [w650] -> _
        shift-left: _ -> [w649]
        shift-right: [w651] -> _
        shift-left: _ -> [w648]
        shift-right: [w647] -> _
        shift-left: _ -> [w645]
        shift-right: [w646] -> _
        shift-left: _ -> [w644]
        shift-right: [w643] -> _
        shift-left: _ -> [w641]
        shift-right: [w642] -> _
        shift-left: _ -> [w640]
        shift-right: [w639] -> _
        shift-left: _ -> [w637]
        shift-right: [w638] -> _
        shift-left: _ -> [w636]
        shift-right: [w634] -> _
        shift-left: _ -> [w632]
        shift-right: [w635] -> _
        shift-left: _ -> [w633]
        shift-right: [w630] -> _
        shift-left: _ -> [w628]
        shift-right: [w631] -> _
        shift-left: _ -> [w629]
        stop <- w699 stop-if-true
        w664 = fxp<+/-,20,5> 0.0 ("fixed-point type")
        n403 = local read "Sample X Stage Displacement (nm)"() -> (w624:fxp<+/-,58,25>)
        n404 = local read "Sample Y Stage Displacement (nm)"() -> (w621:fxp<+/-,58,25>)
        n405 = local read "Sample Z Stage Displacement (nm)"() -> (w618:fxp<+/-,58,25>)
        n406 = local read "Optics Z Stage Displacement (nm)"() -> (w617:fxp<+/-,58,25>)
        n407 = local read "Optics X Stage Displacement (nm)"() -> (w623:fxp<+/-,58,25>)
        n408 = local read "Optics Y Stage Displacement (nm)"() -> (w620:fxp<+/-,58,25>)
        n409 = case shown="\"FPGA Generated Reference\", Default" "Reference Signal Source" {
          tunnel: [w703 w706] -> w627
          tunnel: [w702 w705] -> w626
          tunnel: [w701 w704] -> w625
          frame "FPGA Generated Reference", Default {
            n410 = local read "X Stage Reference (nm)"() -> (w703:fxp<+/-,58,25>)
            n411 = local read "Y Stage Reference (nm)"() -> (w702:fxp<+/-,58,25>)
            n412 = local read "Z Stage Reference (nm)"() -> (w701:fxp<+/-,58,25>)
          }
          frame "External Reference" {
            n413 = local read "X Stage External Reference (nm)"() -> (w706:fxp<+/-,58,25>)
            n414 = local read "Y Stage External Reference (nm)"() -> (w705:fxp<+/-,58,25>)
            n415 = local read "Z Stage External Reference (nm)"() -> (w704:fxp<+/-,58,25>)
          }
        }
        n416 = case shown="\"Optics Stage Only\", Default" "Optics and or Sample Stage" {
          tunnel: w624 -> [_ w718]
          tunnel: w623 -> [w709 w717]
          tunnel: [w709 w716] -> w622
          tunnel: w621 -> [_ w715]
          tunnel: w620 -> [w708 w714]
          tunnel: [w708 w713] -> w619
          tunnel: w618 -> [_ w712]
          tunnel: w617 -> [w707 w711]
          tunnel: [w707 w710] -> w616
          frame "Optics Stage Only", Default {
          }
          frame "Optics and Sample Stage" {
            n417 = Subtract(x=w717, y=w718) -> (x-y=w716:fxp<+/-,59,26>)
            n418 = Subtract(x=w714, y=w715) -> (x-y=w713:fxp<+/-,59,26>)
            n419 = Subtract(x=w711, y=w712) -> (x-y=w710:fxp<+/-,59,26>)
          }
        }
        n420 = call "Loop Timer3"("Count(uSec)"="Controller Time Period (uSec)") -> ()  [unwired: 1 out]
        n421 = case shown="\"Open Loop\", Default" "System Loop Type" {
          tunnel: w622 -> [_ w822]
          tunnel: w627 -> [w734 w823]
          tunnel: [w727 w796] -> w688
          tunnel: [w728 w821] -> w668
          tunnel: [_ w818] -> w686
          tunnel: [_ w817] -> w685
          tunnel: [_ w816] -> w684
          tunnel: [_ w815] -> w683
          tunnel: [_ w814] -> w682
          tunnel: [_ w813] -> w681
          tunnel: [_ w812] -> w680
          tunnel: [_ w811] -> w679
          tunnel: [_ w810] -> w678
          tunnel: w676 -> [_ w809]
          tunnel: w675 -> [_ w808]
          tunnel: w674 -> [_ w807]
          tunnel: w673 -> [_ w806]
          tunnel: w672 -> [_ w805]
          tunnel: w671 -> [_ w804]
          tunnel: w670 -> [_ w803]
          tunnel: w669 -> [_ w802]
          tunnel: w619 -> [_ w800]
          tunnel: w626 -> [w733 w801]
          tunnel: w625 -> [w732 w794]
          tunnel: w616 -> [_ w793]
          tunnel: [w726 w797] -> w687
          tunnel: w677 -> [_ w799]
          tunnel: [_ w789] -> w663
          tunnel: w662 -> [_ w788]
          tunnel: [_ w787] -> w661
          tunnel: w660 -> [_ w786]
          tunnel: [_ w785] -> w659
          tunnel: w658 -> [_ w784]
          tunnel: [_ w778] -> w657
          tunnel: w656 -> [_ w777]
          tunnel: [_ w776] -> w655
          tunnel: w654 -> [_ w775]
          tunnel: [_ w774] -> w653
          tunnel: w652 -> [_ w773]
          tunnel: [_ w767] -> w650
          tunnel: [_ w766] -> w651
          tunnel: w649 -> [_ w765]
          tunnel: w648 -> [_ w764]
          tunnel: [_ w763] -> w647
          tunnel: [_ w762] -> w646
          tunnel: w645 -> [_ w761]
          tunnel: w644 -> [_ w760]
          tunnel: [_ w759] -> w643
          tunnel: [_ w758] -> w642
          tunnel: w641 -> [_ w757]
          tunnel: w640 -> [_ w756]
          tunnel: [_ w755] -> w639
          tunnel: [_ w754] -> w638
          tunnel: w637 -> [_ w753]
          tunnel: w636 -> [_ w752]
          tunnel: [_ w746] -> w635
          tunnel: [_ w745] -> w634
          tunnel: w633 -> [_ w744]
          tunnel: w632 -> [_ w743]
          tunnel: [_ w742] -> w631
          tunnel: [_ w741] -> w630
          tunnel: w629 -> [_ w740]
          tunnel: w628 -> [_ w739]
          frame "Open Loop", Default {
            w725 = fxp<+/-,58,25> 0.0 ("fixed-point type")
            n422 = Multiply(x="X-Stage nm to V Scaling", y="X-Stage Scaling Direction") -> (x*y=w736:fxp<+/-,35,15>)
            n423 = Multiply(x="Y-Stage nm to V Scaling", y="Y-Stage Scaling Direction") -> (x*y=w722:fxp<+/-,35,15>)
            n424 = Multiply(x="Z-Stage nm to V Scaling", y="Z-Stage Scaling Direction") -> (x*y=w721:fxp<+/-,35,15>)
            n425 = Multiply(x=w734, y=w736) -> (x*y=w731:fxp<+/-,64,38>)
            n426 = Multiply(x=w733, y=w722) -> (x*y=w730:fxp<+/-,64,38>)
            n427 = Multiply(x=w732, y=w721) -> (x*y=w729:fxp<+/-,64,38>)
            n428 = To Fixed-Point(fixed-point type=w725, number=w731) -> (fixed-point=w728:fxp<+/-,58,25>)
            n429 = To Fixed-Point(fixed-point type=w725, number=w730) -> (fixed-point=w727:fxp<+/-,58,25>)
            n430 = To Fixed-Point(fixed-point type=w725, number=w729) -> (fixed-point=w726:fxp<+/-,58,25>)
          }
          frame "Closed Loop" {
            w738 = fxp<+/-,58,25> 0.0 ("fixed-point type")
            w790 = fxp<+/-,58,25> 0.0 ("fixed-point type")
            n431 = Subtract(x=w823, y=w822) -> (x-y=w827:fxp<+/-,60,27>)
            n432 = Subtract(x=w801, y=w800) -> (x-y=w826:fxp<+/-,60,27>)
            n433 = Subtract(x=w794, y=w793) -> (x-y=w795:fxp<+/-,60,27>)
            n434 = To Fixed-Point(fixed-point type=w738, number=w827) -> (fixed-point=w825:fxp<+/-,58,25>)
            n435 = To Fixed-Point(fixed-point type=w738, number=w826) -> (fixed-point=w824:fxp<+/-,58,25>)
            n436 = To Fixed-Point(fixed-point type=w738, number=w795) -> (fixed-point=w792:fxp<+/-,58,25>)
            n437 = for {
              N: 9 -> [_]
              shift-right: [w1062] -> w780
              shift-left: _ -> [w1060]
              shift-right: [w1059] -> w770
              shift-left: _ -> [w1057]
              tunnel: [w1050] -> w818
              shift-right: [w1049] -> _
              shift-left: _ -> [w1045]
              tunnel: [w1048] -> w817
              shift-right: [w1047] -> _
              shift-left: _ -> [w1043]
              tunnel: w799 -> [w1040]
              tunnel: w809 -> [w1039]
              tunnel: [w1038] -> w815
              shift-right: [w1037] -> _
              shift-left: _ -> [w1030]
              tunnel: [w1036] -> w814
              shift-right: [w1035] -> _
              shift-left: _ -> [w1029]
              tunnel: [w1034] -> w812
              tunnel: [w1033] -> w811
              shift-right: [w1032] -> _
              shift-left: _ -> [w1028]
              shift-right: [w1031] -> _
              shift-left: _ -> [w1017]
              tunnel: w807 -> [w1027]
              tunnel: w806 -> [w1026]
              tunnel: w804 -> [w1025]
              tunnel: w803 -> [w1024]
              tunnel: w825 -> [w1016]
              tunnel: w824 -> [w1013]
              shift-right: [w1012] -> w750
              shift-left: _ -> [w1008]
              tunnel: [w1003] -> w816
              tunnel: [w1002] -> w813
              tunnel: [w1001] -> w810
              shift-right: [w1000] -> _
              shift-left: _ -> [w996]
              shift-right: [w999] -> _
              shift-left: _ -> [w994]
              shift-right: [w998] -> _
              shift-left: _ -> [w992]
              tunnel: w808 -> [w991]
              tunnel: w802 -> [w990]
              tunnel: w805 -> [w989]
              tunnel: w792 -> [w985]
              shift-right: [w982] -> w782
              shift-left: _ -> [w980]
              tunnel: [w978] -> w789
              shift-right: [w979] -> _
              shift-left: _ -> [w974]
              tunnel: w788 -> [w973]
              tunnel: [w970] -> w787
              shift-right: [w969] -> _
              shift-left: _ -> [w967]
              tunnel: w786 -> [w968]
              tunnel: [w963] -> w785
              shift-right: [w962] -> _
              shift-left: _ -> [w960]
              tunnel: w784 -> [w959]
              shift-right: [w958] -> w783
              shift-left: _ -> [w955]
              tunnel: [w951] -> w778
              shift-right: [w952] -> _
              shift-left: _ -> [w948]
              tunnel: w777 -> [w950]
              tunnel: [w945] -> w776
              shift-right: [w944] -> _
              shift-left: _ -> [w941]
              tunnel: w775 -> [w943]
              tunnel: [w938] -> w774
              shift-right: [w937] -> _
              shift-left: _ -> [w935]
              tunnel: w773 -> [w934]
              shift-right: [w930] -> w769
              shift-left: _ -> [w927]
              shift-right: [w929] -> w771
              shift-left: _ -> [w925]
              tunnel: [w920] -> w767
              shift-right: [w919] -> _
              shift-left: _ -> [w913]
              tunnel: [w918] -> w766
              shift-right: [w917] -> _
              shift-left: _ -> [w911]
              tunnel: w765 -> [w910]
              tunnel: w764 -> [w909]
              tunnel: [w907] -> w763
              shift-right: [w906] -> _
              shift-left: _ -> [w899]
              tunnel: [w903] -> w762
              shift-right: [w902] -> _
              shift-left: _ -> [w897]
              tunnel: w761 -> [w896]
              tunnel: w760 -> [w895]
              tunnel: [w892] -> w759
              tunnel: [w890] -> w758
              shift-right: [w891] -> _
              shift-left: _ -> [w883]
              shift-right: [w889] -> _
              shift-left: _ -> [w885]
              tunnel: w757 -> [w882]
              tunnel: w756 -> [w881]
              tunnel: [w876] -> w755
              tunnel: [w875] -> w754
              shift-right: [w874] -> _
              shift-left: _ -> [w871]
              shift-right: [w873] -> _
              shift-left: _ -> [w869]
              tunnel: w753 -> [w868]
              tunnel: w752 -> [w867]
              shift-right: [w864] -> w748
              shift-left: _ -> [w861]
              shift-right: [w863] -> w749
              shift-left: _ -> [w859]
              tunnel: [w854] -> w746
              tunnel: [w853] -> w745
              shift-right: [w852] -> _
              shift-left: _ -> [w847]
              shift-right: [w851] -> _
              shift-left: _ -> [w845]
              tunnel: w744 -> [w844]
              tunnel: w743 -> [w843]
              shift-right: [w838] -> _
              shift-left: _ -> [w833]
              shift-right: [w837] -> _
              shift-left: _ -> [w831]
              tunnel: [w836] -> w742
              tunnel: [w835] -> w741
              tunnel: w740 -> [w830]
              tunnel: w739 -> [w829]
              i -> [w1068]
              # "ez"
              # "ey"
              # "ex"
              n438 = Add(x=1, y=w1068) -> (x+y=w1065:i32)
              n439 = flat-sequence {
                tunnel: [w1202] -> w1082
                tunnel: [w1201] -> w1081
                tunnel: [w1200] -> w1080
                tunnel: [w1199] -> w1079
                tunnel: [w1198] -> w1078
                tunnel: [w1197] -> w1077
                tunnel: [w1196] -> w1076
                tunnel: [w1195] -> w1075
                tunnel: w1065 -> [w1203]
                tunnel: [w1181] -> w1070
                tunnel: [w1194] -> w1061
                tunnel: w1060 -> [w1194]
                tunnel: [w1193] -> w1058
                tunnel: w1057 -> [w1193]
                tunnel: [w1192] -> w1046
                tunnel: w1045 -> [w1192]
                tunnel: [w1119] -> w1044
                tunnel: w1043 -> [w1119]
                tunnel: w1040 -> [w1183]
                tunnel: w1039 -> [w1184]
                tunnel: w1030 -> [w1191]
                tunnel: w1029 -> [w1190]
                tunnel: w1028 -> [w1189]
                tunnel: w1027 -> [w1185]
                tunnel: w1026 -> [w1186]
                tunnel: w1025 -> [w1187]
                tunnel: w1024 -> [w1188]
                tunnel: w1017 -> [w1182]
                tunnel: [w1191] -> w1023
                tunnel: [w1190] -> w1022
                tunnel: [w1189] -> w1021
                tunnel: w1016 -> [w1157]
                tunnel: [w1182] -> w1015
                tunnel: w1013 -> [w1179]
                tunnel: [w1180] -> w1009
                tunnel: w1008 -> [w1180]
                tunnel: [w1178] -> w997
                tunnel: w996 -> [w1178]
                tunnel: [w1177] -> w995
                tunnel: w994 -> [w1177]
                tunnel: [w1176] -> w993
                tunnel: w992 -> [w1176]
                tunnel: w991 -> [w1173]
                tunnel: w990 -> [w1175]
                tunnel: w989 -> [w1174]
                tunnel: w985 -> [w1156]
                tunnel: [w1150] -> w981
                tunnel: w980 -> [w1150]
                tunnel: [w1149] -> w975
                tunnel: w974 -> [w1149]
                tunnel: w973 -> [w1148]
                tunnel: w968 -> [w1146]
                tunnel: w967 -> [w1147]
                tunnel: [w1147] -> w966
                tunnel: [w1145] -> w961
                tunnel: w960 -> [w1145]
                tunnel: w959 -> [w1144]
                tunnel: [w1138] -> w956
                tunnel: w955 -> [w1138]
                tunnel: w950 -> [w1136]
                tunnel: [w1137] -> w949
                tunnel: w948 -> [w1137]
                tunnel: w943 -> [w1134]
                tunnel: [w1135] -> w942
                tunnel: w941 -> [w1135]
                tunnel: [w1133] -> w936
                tunnel: w935 -> [w1133]
                tunnel: w934 -> [w1132]
                tunnel: [w1121] -> w928
                tunnel: w927 -> [w1121]
                tunnel: [w1120] -> w926
                tunnel: w925 -> [w1120]
                tunnel: [w1118] -> w914
                tunnel: w913 -> [w1118]
                tunnel: [w1117] -> w912
                tunnel: w911 -> [w1117]
                tunnel: w910 -> [w1115]
                tunnel: w909 -> [w1116]
                tunnel: [w1114] -> w900
                tunnel: w899 -> [w1114]
                tunnel: [w1113] -> w898
                tunnel: w897 -> [w1113]
                tunnel: w896 -> [w1111]
                tunnel: w895 -> [w1112]
                tunnel: [w1110] -> w886
                tunnel: w885 -> [w1110]
                tunnel: [w1109] -> w884
                tunnel: w883 -> [w1109]
                tunnel: w882 -> [w1108]
                tunnel: w881 -> [w1107]
                tunnel: [w1106] -> w872
                tunnel: w871 -> [w1106]
                tunnel: [w1105] -> w870
                tunnel: w869 -> [w1105]
                tunnel: w868 -> [w1104]
                tunnel: w867 -> [w1103]
                tunnel: [w1092] -> w862
                tunnel: w861 -> [w1092]
                tunnel: [w1091] -> w860
                tunnel: w859 -> [w1091]
                tunnel: [w1090] -> w848
                tunnel: w847 -> [w1090]
                tunnel: [w1089] -> w846
                tunnel: w845 -> [w1089]
                tunnel: w844 -> [w1088]
                tunnel: w843 -> [w1087]
                tunnel: [w1086] -> w834
                tunnel: w833 -> [w1086]
                tunnel: [w1085] -> w832
                tunnel: w831 -> [w1085]
                tunnel: w830 -> [w1083]
                tunnel: w829 -> [w1084]
                tunnel: w1082 -> [w1333]
                tunnel: w1081 -> [w1332]
                tunnel: w1080 -> [w1331]
                tunnel: w1079 -> [w1330]
                tunnel: w1078 -> [w1329]
                tunnel: w1077 -> [w1328]
                tunnel: w1076 -> [w1327]
                tunnel: w1075 -> [w1326]
                tunnel: [w1295] -> w1074
                tunnel: [w1296] -> w1073
                tunnel: [w1290] -> w1072
                tunnel: [w1289] -> w1071
                tunnel: w1070 -> [w1313]
                tunnel: [w1295] -> w1067
                tunnel: [w1295] -> w1066
                tunnel: [w1324] -> w1064
                tunnel: [w1325] -> w1063
                tunnel: w1061 -> [w1325]
                tunnel: w1058 -> [w1324]
                tunnel: [w1296] -> w1056
                tunnel: [w1296] -> w1055
                tunnel: [w1290] -> w1054
                tunnel: [w1290] -> w1053
                tunnel: [w1289] -> w1052
                tunnel: [w1289] -> w1051
                tunnel: w1046 -> [w1323]
                tunnel: w1044 -> [w1322]
                tunnel: [w1323] -> w1042
                tunnel: [w1322] -> w1041
                tunnel: w1023 -> [w1321]
                tunnel: w1022 -> [w1320]
                tunnel: w1021 -> [w1319]
                tunnel: [w1321] -> w1020
                tunnel: [w1320] -> w1019
                tunnel: [w1319] -> w1018
                tunnel: w1015 -> [w1318]
                tunnel: [w1318] -> w1014
                tunnel: [w1295] -> w1011
                tunnel: [w1295] -> w1010
                tunnel: w1009 -> [w1317]
                tunnel: [w1317] -> w1007
                tunnel: [w1296] -> w1006
                tunnel: [w1290] -> w1005
                tunnel: [w1289] -> w1004
                tunnel: w997 -> [w1316]
                tunnel: w995 -> [w1315]
                tunnel: w993 -> [w1314]
                tunnel: [w1316] -> w988
                tunnel: [w1315] -> w987
                tunnel: [w1314] -> w986
                tunnel: [w1295] -> w984
                tunnel: [w1312] -> w983
                tunnel: w981 -> [w1312]
                tunnel: [w1296] -> w977
                tunnel: [w1311] -> w976
                tunnel: w975 -> [w1311]
                tunnel: [w1290] -> w972
                tunnel: [w1310] -> w971
                tunnel: w966 -> [w1310]
                tunnel: [w1289] -> w965
                tunnel: [w1309] -> w964
                tunnel: w961 -> [w1309]
                tunnel: [w1295] -> w957
                tunnel: w956 -> [w1308]
                tunnel: [w1308] -> w954
                tunnel: [w1296] -> w953
                tunnel: w949 -> [w1307]
                tunnel: [w1307] -> w947
                tunnel: [w1290] -> w946
                tunnel: w942 -> [w1306]
                tunnel: [w1306] -> w940
                tunnel: [w1289] -> w939
                tunnel: w936 -> [w1305]
                tunnel: [w1305] -> w933
                tunnel: [w1295] -> w932
                tunnel: [w1295] -> w931
                tunnel: w928 -> [w1304]
                tunnel: w926 -> [w1303]
                tunnel: [w1304] -> w924
                tunnel: [w1303] -> w923
                tunnel: [w1296] -> w922
                tunnel: [w1296] -> w921
                tunnel: [w1301] -> w916
                tunnel: [w1302] -> w915
                tunnel: w914 -> [w1302]
                tunnel: w912 -> [w1301]
                tunnel: [w1290] -> w908
                tunnel: [w1300] -> w905
                tunnel: [w1290] -> w904
                tunnel: [w1299] -> w901
                tunnel: w900 -> [w1300]
                tunnel: w898 -> [w1299]
                tunnel: [w1289] -> w894
                tunnel: [w1289] -> w893
                tunnel: [w1298] -> w888
                tunnel: [w1297] -> w887
                tunnel: w886 -> [w1297]
                tunnel: w884 -> [w1298]
                tunnel: [w1296] -> w880
                tunnel: [w1296] -> w879
                tunnel: [w1292] -> w878
                tunnel: [w1291] -> w877
                tunnel: w872 -> [w1292]
                tunnel: w870 -> [w1291]
                tunnel: [w1295] -> w866
                tunnel: [w1295] -> w865
                tunnel: w862 -> [w1294]
                tunnel: w860 -> [w1293]
                tunnel: [w1294] -> w858
                tunnel: [w1293] -> w857
                tunnel: [w1290] -> w856
                tunnel: [w1290] -> w855
                tunnel: [w1288] -> w850
                tunnel: [w1287] -> w849
                tunnel: w848 -> [w1288]
                tunnel: w846 -> [w1287]
                tunnel: [w1289] -> w842
                tunnel: [w1289] -> w841
                tunnel: [w1286] -> w840
                tunnel: [w1285] -> w839
                tunnel: w834 -> [w1286]
                tunnel: w832 -> [w1285]
                tunnel: w1074 -> [_]
                tunnel: w1073 -> [_]
                tunnel: w1072 -> [_]
                tunnel: w1071 -> [_]
                tunnel: w1067 -> [w1536]
                tunnel: w1066 -> [w1535]
                tunnel: w1065 -> [w1364]
                tunnel: w1064 -> [w1534]
                tunnel: w1063 -> [w1533]
                tunnel: [w1483] -> w1062
                tunnel: [w1482] -> w1059
                tunnel: w1056 -> [w1520]
                tunnel: w1055 -> [w1519]
                tunnel: w1054 -> [w1518]
                tunnel: w1053 -> [w1517]
                tunnel: w1052 -> [w1516]
                tunnel: w1051 -> [w1515]
                tunnel: [w1514] -> w1050
                tunnel: [w1514] -> w1049
                tunnel: [w1513] -> w1048
                tunnel: [w1513] -> w1047
                tunnel: w1042 -> [w1512]
                tunnel: w1041 -> [w1511]
                tunnel: [w1510] -> w1038
                tunnel: [w1510] -> w1037
                tunnel: [w1509] -> w1036
                tunnel: [w1509] -> w1035
                tunnel: [w1508] -> w1034
                tunnel: [w1507] -> w1033
                tunnel: [w1508] -> w1032
                tunnel: [w1507] -> w1031
                tunnel: w1020 -> [w1506]
                tunnel: w1019 -> [w1505]
                tunnel: w1018 -> [w1504]
                tunnel: w1014 -> [w1503]
                tunnel: [w1481] -> w1012
                tunnel: w1011 -> [w1500]
                tunnel: w1010 -> [_]
                tunnel: w1007 -> [w1499]
                tunnel: w1006 -> [w1492]
                tunnel: w1005 -> [w1491]
                tunnel: w1004 -> [w1490]
                tunnel: [w1489] -> w1003
                tunnel: [w1488] -> w1002
                tunnel: [w1487] -> w1001
                tunnel: [w1489] -> w1000
                tunnel: [w1488] -> w999
                tunnel: [w1487] -> w998
                tunnel: w988 -> [w1486]
                tunnel: w987 -> [w1485]
                tunnel: w986 -> [w1484]
                tunnel: w984 -> [w1478]
                tunnel: [w1477] -> w982
                tunnel: w983 -> [w1476]
                tunnel: [w1473] -> w978
                tunnel: [w1473] -> w979
                tunnel: w977 -> [w1472]
                tunnel: w976 -> [w1471]
                tunnel: w972 -> [w1468]
                tunnel: w971 -> [w1467]
                tunnel: [w1466] -> w970
                tunnel: [w1466] -> w969
                tunnel: w965 -> [w1463]
                tunnel: w964 -> [w1462]
                tunnel: [w1461] -> w963
                tunnel: [w1461] -> w962
                tunnel: [w1458] -> w958
                tunnel: w957 -> [w1457]
                tunnel: w954 -> [w1456]
                tunnel: w953 -> [w1453]
                tunnel: [w1452] -> w951
                tunnel: [w1452] -> w952
                tunnel: w947 -> [w1451]
                tunnel: [w1448] -> w945
                tunnel: [w1448] -> w944
                tunnel: w946 -> [w1447]
                tunnel: w940 -> [w1446]
                tunnel: w939 -> [w1443]
                tunnel: [w1442] -> w938
                tunnel: [w1442] -> w937
                tunnel: w933 -> [w1441]
                tunnel: w932 -> [w1436]
                tunnel: w931 -> [w1435]
                tunnel: [w1434] -> w930
                tunnel: [w1433] -> w929
                tunnel: w924 -> [w1432]
                tunnel: w923 -> [w1431]
                tunnel: w922 -> [w1426]
                tunnel: w921 -> [w1425]
                tunnel: [w1424] -> w920
                tunnel: [w1424] -> w919
                tunnel: [w1423] -> w918
                tunnel: [w1423] -> w917
                tunnel: w916 -> [w1422]
                tunnel: w915 -> [w1421]
                tunnel: w908 -> [w1418]
                tunnel: [w1417] -> w907
                tunnel: [w1417] -> w906
                tunnel: w905 -> [w1416]
                tunnel: w904 -> [w1413]
                tunnel: [w1412] -> w903
                tunnel: [w1412] -> w902
                tunnel: w901 -> [w1411]
                tunnel: w894 -> [w1406]
                tunnel: w893 -> [w1405]
                tunnel: [w1404] -> w892
                tunnel: [w1404] -> w891
                tunnel: [w1403] -> w890
                tunnel: [w1403] -> w889
                tunnel: w888 -> [w1402]
                tunnel: w887 -> [w1401]
                tunnel: w880 -> [w1396]
                tunnel: w879 -> [w1395]
                tunnel: w878 -> [w1394]
                tunnel: w877 -> [w1393]
                tunnel: [w1392] -> w876
                tunnel: [w1392] -> w874
                tunnel: [w1391] -> w875
                tunnel: [w1391] -> w873
                tunnel: w866 -> [w1386]
                tunnel: w865 -> [w1385]
                tunnel: [w1384] -> w864
                tunnel: [w1383] -> w863
                tunnel: w858 -> [w1382]
                tunnel: w857 -> [w1381]
                tunnel: w856 -> [w1376]
                tunnel: w855 -> [w1375]
                tunnel: [w1374] -> w854
                tunnel: [w1374] -> w852
                tunnel: [w1373] -> w853
                tunnel: [w1373] -> w851
                tunnel: w850 -> [w1372]
                tunnel: w849 -> [w1371]
                tunnel: w842 -> [w1366]
                tunnel: w841 -> [w1365]
                tunnel: w840 -> [w1363]
                tunnel: w839 -> [w1362]
                tunnel: [w1361] -> w836
                tunnel: [w1361] -> w838
                tunnel: [w1360] -> w835
                tunnel: [w1360] -> w837
                frame #0 {
                  n440 = case shown="1, Default" w1203 {
                    tunnel: [w1212 w1221 w1225 w1239 w1244 w1252 w1262 w1267 w1280] -> w1199
                    tunnel: [w1211 w1217 w1226 w1235 w1245 w1253 w1258 w1268 w1281] -> w1198
                    tunnel: [w1210 w1218 w1227 w1236 w1246 w1254 w1259 w1269 w1282] -> w1197
                    tunnel: [w1208 w1219 w1228 w1237 w1247 w1255 w1260 w1270 w1283] -> w1196
                    tunnel: [w1209 w1220 w1229 w1238 w1248 w1256 w1261 w1271 w1284] -> w1195
                    tunnel: "sos gain SF Controller xx1" -> [w1212 _ _ _ _ _ _ _ _]
                    tunnel: "-a01(2) xx1" -> [w1211 _ _ _ _ _ _ _ _]
                    tunnel: "-a02(2) xx1" -> [w1210 _ _ _ _ _ _ _ _]
                    tunnel: "b01(2) xx1" -> [w1208 _ _ _ _ _ _ _ _]
                    tunnel: "b02(2) xx1" -> [w1209 _ _ _ _ _ _ _ _]
                    tunnel: "sos gain SF Controller yy1" -> [_ _ _ _ w1244 _ _ _ _]
                    tunnel: "-a01(2) yy1" -> [_ _ _ _ w1245 _ _ _ _]
                    tunnel: "-a02(2) yy1" -> [_ _ _ _ w1246 _ _ _ _]
                    tunnel: "b01(2) yy1" -> [_ _ _ _ w1247 _ _ _ _]
                    tunnel: "b02(2) yy1" -> [_ _ _ _ w1248 _ _ _ _]
                    tunnel: [w1205 w1214 w1224 w1233 w1243 w1251 w1266 w1275 w1279] -> w1200
                    tunnel: [w1206 w1215 w1223 w1232 w1242 w1250 w1265 w1274 w1278] -> w1201
                    tunnel: [w1207 w1216 w1222 w1231 w1241 w1249 w1264 w1273 w1277] -> w1202
                    tunnel: w1183 -> [w1207 _ _ _ _ _ _ _ _]
                    tunnel: w1184 -> [_ _ _ _ w1241 _ _ _ _]
                    tunnel: w1185 -> [w1206 _ _ _ _ _ _ _ _]
                    tunnel: w1186 -> [_ _ _ _ w1242 _ _ _ _]
                    tunnel: w1187 -> [w1205 _ _ _ _ _ _ _ _]
                    tunnel: w1188 -> [_ _ _ _ w1243 _ _ _ _]
                    tunnel: [w1204 w1213 w1230 w1234 w1240 w1257 w1263 w1272 w1276] -> w1181
                    tunnel: w1157 -> [w1204 _ _ w1234 _ _ w1263 _ _]
                    tunnel: "sos gain SF Controller zz1" -> [_ _ _ _ _ _ _ _ w1280]
                    tunnel: "-a01(2) zz1" -> [_ _ _ _ _ _ _ _ w1281]
                    tunnel: "-a02(2) zz1" -> [_ _ _ _ _ _ _ _ w1282]
                    tunnel: "b01(2) zz1" -> [_ _ _ _ _ _ _ _ w1283]
                    tunnel: "b02(2) zz1" -> [_ _ _ _ _ _ _ _ w1284]
                    tunnel: w1179 -> [_ w1213 _ _ w1240 _ _ w1272 _]
                    tunnel: w1175 -> [_ _ _ _ _ _ _ _ w1279]
                    tunnel: w1174 -> [_ _ _ _ _ _ _ _ w1278]
                    tunnel: w1173 -> [_ _ _ _ _ _ _ _ w1277]
                    tunnel: w1156 -> [_ _ w1230 _ _ w1257 _ _ w1276]
                    tunnel: "sos gain SF Controller yx1" -> [_ w1221 _ _ _ _ _ _ _]
                    tunnel: "-a01(2) yx1" -> [_ w1217 _ _ _ _ _ _ _]
                    tunnel: "-a02(2) yx1" -> [_ w1218 _ _ _ _ _ _ _]
                    tunnel: "b01(2) yx1" -> [_ w1219 _ _ _ _ _ _ _]
                    tunnel: "b02(2) yx1" -> [_ w1220 _ _ _ _ _ _ _]
                    tunnel: w1148 -> [_ w1216 _ _ _ _ _ _ _]
                    tunnel: w1146 -> [_ w1215 _ _ _ _ _ _ _]
                    tunnel: w1144 -> [_ w1214 _ _ _ _ _ _ _]
                    tunnel: "sos gain SF Controller zx1" -> [_ _ w1225 _ _ _ _ _ _]
                    tunnel: "-a01(2) zx1" -> [_ _ w1226 _ _ _ _ _ _]
                    tunnel: "-a02(2) zx1" -> [_ _ w1227 _ _ _ _ _ _]
                    tunnel: "b01(2) zx1" -> [_ _ w1228 _ _ _ _ _ _]
                    tunnel: "b02(2) zx1" -> [_ _ w1229 _ _ _ _ _ _]
                    tunnel: w1132 -> [_ _ w1224 _ _ _ _ _ _]
                    tunnel: w1134 -> [_ _ w1223 _ _ _ _ _ _]
                    tunnel: w1136 -> [_ _ w1222 _ _ _ _ _ _]
                    tunnel: "sos gain SF Controller xy1" -> [_ _ _ w1239 _ _ _ _ _]
                    tunnel: "-a01(2) xy1" -> [_ _ _ w1235 _ _ _ _ _]
                    tunnel: "-a02(2) xy1" -> [_ _ _ w1236 _ _ _ _ _]
                    tunnel: "b01(2) xy1" -> [_ _ _ w1237 _ _ _ _ _]
                    tunnel: "b02(2) xy1" -> [_ _ _ w1238 _ _ _ _ _]
                    tunnel: "sos gain SF Controller zy1" -> [_ _ _ _ _ w1252 _ _ _]
                    tunnel: "-a01(2) zy1" -> [_ _ _ _ _ w1253 _ _ _]
                    tunnel: "-a02(2) zy1" -> [_ _ _ _ _ w1254 _ _ _]
                    tunnel: "b01(2) zy1" -> [_ _ _ _ _ w1255 _ _ _]
                    tunnel: "b02(2) zy1" -> [_ _ _ _ _ w1256 _ _ _]
                    tunnel: w1107 -> [_ _ _ _ _ w1251 _ _ _]
                    tunnel: w1112 -> [_ _ _ _ _ w1250 _ _ _]
                    tunnel: w1116 -> [_ _ _ _ _ w1249 _ _ _]
                    tunnel: w1108 -> [_ _ _ w1233 _ _ _ _ _]
                    tunnel: w1111 -> [_ _ _ w1232 _ _ _ _ _]
                    tunnel: w1115 -> [_ _ _ w1231 _ _ _ _ _]
                    tunnel: w1084 -> [_ _ _ _ _ _ _ w1275 _]
                    tunnel: w1083 -> [_ _ _ _ _ _ w1266 _ _]
                    tunnel: w1087 -> [_ _ _ _ _ _ _ w1274 _]
                    tunnel: w1088 -> [_ _ _ _ _ _ w1265 _ _]
                    tunnel: w1103 -> [_ _ _ _ _ _ _ w1273 _]
                    tunnel: w1104 -> [_ _ _ _ _ _ w1264 _ _]
                    tunnel: "sos gain SF Controller xz1" -> [_ _ _ _ _ _ w1262 _ _]
                    tunnel: "-a01(2) xz1" -> [_ _ _ _ _ _ w1258 _ _]
                    tunnel: "-a02(2) xz1" -> [_ _ _ _ _ _ w1259 _ _]
                    tunnel: "b01(2) xz1" -> [_ _ _ _ _ _ w1260 _ _]
                    tunnel: "b02(2) xz1" -> [_ _ _ _ _ _ w1261 _ _]
                    tunnel: "sos gain SF Controller yz1" -> [_ _ _ _ _ _ _ w1267 _]
                    tunnel: "-a01(2) yz1" -> [_ _ _ _ _ _ _ w1268 _]
                    tunnel: "-a02(2) yz1" -> [_ _ _ _ _ _ _ w1269 _]
                    tunnel: "b01(2) yz1" -> [_ _ _ _ _ _ _ w1270 _]
                    tunnel: "b02(2) yz1" -> [_ _ _ _ _ _ _ w1271 _]
                    frame 1, Default {
                    }
                    frame 2 {
                    }
                    frame 3 {
                    }
                    frame 4 {
                    }
                    frame 5 {
                    }
                    frame 6 {
                    }
                    frame 7 {
                    }
                    frame 8 {
                    }
                    frame 9 {
                    }
                  }
                }
                frame #1 {
                  n441 = Multiply(x=w1313, y=w1330) -> (x*y=w1334:fxp<+/-,64,34>)
                  n442 = To Fixed-Point(number=w1334) -> (fixed-point=w1335:fxp<+/-,58,25>)  [unwired: 1 in]
                  n443 = for {
                    tunnel: w1329 -> [w1351] mode=indexing
                    tunnel: w1326 -> [w1348] mode=indexing
                    shift-right: [w1353] -> w1295
                    shift-left: w1335 -> [w1352]
                    tunnel: w1328 -> [w1350] mode=indexing
                    tunnel: w1327 -> [w1349] mode=indexing
                    tunnel: [w1340] -> w1296 mode=indexing
                    tunnel: w1333 -> [w1346] mode=indexing
                    tunnel: [w1343] -> w1290 mode=indexing
                    tunnel: w1332 -> [w1336] mode=indexing
                    tunnel: [w1336] -> w1289 mode=indexing
                    tunnel: w1331 -> [w1344] mode=indexing
                    n444 = To Fixed-Point(number=w1346) -> (fixed-point=w1359:fxp<+/-,58,25>)  [unwired: 1 in]
                    n445 = Add(x=w1352, y=w1359) -> (x+y=w1345:fxp<+/-,59,26>)
                    n446 = To Fixed-Point(number=w1345) -> (fixed-point=w1343:fxp<+/-,58,25>)  [unwired: 1 in]
                    n447 = Multiply(x=w1343, y=w1351) -> (x*y=w1358:fxp<+/-,64,34>)
                    n448 = To Fixed-Point(number=w1358) -> (fixed-point=w1339:fxp<+/-,58,25>)  [unwired: 1 in]
                    n449 = Multiply(x=w1336, y=w1350) -> (x*y=w1354:fxp<+/-,64,34>)
                    n450 = To Fixed-Point(number=w1354) -> (fixed-point=w1338:fxp<+/-,58,25>)  [unwired: 1 in]
                    n451 = Add(x=w1339, y=w1338) -> (x+y=w1347:fxp<+/-,59,26>)
                    n452 = To Fixed-Point(number=w1347) -> (fixed-point=w1340:fxp<+/-,58,25>)  [unwired: 1 in]
                    n453 = Multiply(x=w1336, y=w1349) -> (x*y=w1355:fxp<+/-,64,34>)
                    n454 = Multiply(x=w1344, y=w1348) -> (x*y=w1357:fxp<+/-,64,34>)
                    n455 = To Fixed-Point(number=w1355) -> (fixed-point=w1341:fxp<+/-,58,25>)  [unwired: 1 in]
                    n456 = To Fixed-Point(number=w1357) -> (fixed-point=w1337:fxp<+/-,58,25>)  [unwired: 1 in]
                    n457 = Add(x=w1341, y=w1337) -> (x+y=w1356:fxp<+/-,59,26>)
                    n458 = To Fixed-Point(number=w1356) -> (fixed-point=w1342:fxp<+/-,58,25>)  [unwired: 1 in]
                    n459 = Add(x=w1343, y=w1342) -> (x+y=w1353:fxp<+/-,58,25>)
                  }
                }
                frame #2 {
                  n460 = Equal?(x=6, y=w1364) -> (x = y?=w1437:bool)
                  n461 = Equal?(x=5, y=w1364) -> (x = y?=w1537:bool)
                  n462 = Equal?(x=1, y=w1364) -> (x = y?=w1539:bool)
                  n463 = Equal?(x=9, y=w1364) -> (x = y?=w1501:bool)
                  n464 = Equal?(x=2, y=w1364) -> (x = y?=w1479:bool)
                  n465 = Equal?(x=4, y=w1364) -> (x = y?=w1439:bool)
                  n466 = Equal?(x=7, y=w1364) -> (x = y?=w1387:bool)
                  n467 = Equal?(x=3, y=w1364) -> (x = y?=w1459:bool)
                  n468 = Equal?(x=8, y=w1364) -> (x = y?=w1389:bool)
                  n469 = Equal?(x=6, y=w1364) -> (x = y?=w1407:bool)
                  n470 = Equal?(x=5, y=w1364) -> (x = y?=w1529:bool)
                  n471 = Equal?(x=9, y=w1364) -> (x = y?=w1497:bool)
                  n472 = Equal?(x=5, y=w1364) -> (x = y?=w1525:bool)
                  n473 = Equal?(x=6, y=w1364) -> (x = y?=w1414:bool)
                  n474 = Equal?(x=4, y=w1364) -> (x = y?=w1409:bool)
                  n475 = Equal?(x=5, y=w1364) -> (x = y?=w1521:bool)
                  n476 = Equal?(x=7, y=w1364) -> (x = y?=w1369:bool)
                  n477 = Equal?(x=9, y=w1364) -> (x = y?=w1493:bool)
                  n478 = Equal?(x=1, y=w1364) -> (x = y?=w1531:bool)
                  n479 = Equal?(x=6, y=w1364) -> (x = y?=w1427:bool)
                  n480 = Equal?(x=1, y=w1364) -> (x = y?=w1527:bool)
                  n481 = Equal?(x=2, y=w1364) -> (x = y?=w1469:bool)
                  n482 = Equal?(x=4, y=w1364) -> (x = y?=w1419:bool)
                  n483 = Equal?(x=9, y=w1364) -> (x = y?=w1495:bool)
                  n484 = Equal?(x=1, y=w1364) -> (x = y?=w1523:bool)
                  n485 = Equal?(x=2, y=w1364) -> (x = y?=w1474:bool)
                  n486 = Equal?(x=7, y=w1364) -> (x = y?=w1399:bool)
                  n487 = Equal?(x=8, y=w1364) -> (x = y?=w1397:bool)
                  n488 = Equal?(x=2, y=w1364) -> (x = y?=w1464:bool)
                  n489 = Equal?(x=8, y=w1364) -> (x = y?=w1367:bool)
                  n490 = Equal?(x=4, y=w1364) -> (x = y?=w1429:bool)
                  n491 = Equal?(x=3, y=w1364) -> (x = y?=w1449:bool)
                  n492 = Equal?(x=3, y=w1364) -> (x = y?=w1444:bool)
                  n493 = Equal?(x=7, y=w1364) -> (x = y?=w1379:bool)
                  n494 = Equal?(x=8, y=w1364) -> (x = y?=w1377:bool)
                  n495 = Equal?(x=3, y=w1364) -> (x = y?=w1454:bool)
                  n496 = Select(t=w1435, s=w1437, f=w1431) -> (s? t:f=w1433:fxp<+/-,58,25>)
                  "Kzy Output, Kzy*ez (V)" <- w1433
                  n497 = Select(t=w1535, s=w1537, f=w1534) -> (s? t:f=w1482:fxp<+/-,58,25>)
                  "Kyy Output, Kyy*ey (V)" <- w1482
                  n498 = Select(t=w1536, s=w1539, f=w1533) -> (s? t:f=w1483:fxp<+/-,58,25>)
                  "Kxx Output, Kxx*ex (V)" <- w1483
                  n499 = Select(t=w1500, s=w1501, f=w1499) -> (s? t:f=w1481:fxp<+/-,58,25>)
                  "Kzz Output, Kzz*ez (V)" <- w1481
                  n500 = Select(t=w1436, s=w1439, f=w1432) -> (s? t:f=w1434:fxp<+/-,58,25>)
                  "Kxy Output, Kxy*ex (V)" <- w1434
                  n501 = Select(t=w1386, s=w1387, f=w1382) -> (s? t:f=w1384:fxp<+/-,58,25>)
                  "Kxz Output, Kxz*ex (V)" <- w1384
                  n502 = Select(t=w1478, s=w1479, f=w1476) -> (s? t:f=w1477:fxp<+/-,58,25>)
                  "Kyx Output, Kyx*ey (V)" <- w1477
                  n503 = Select(t=w1385, s=w1389, f=w1381) -> (s? t:f=w1383:fxp<+/-,58,25>)
                  "Kyz Output, Kyz*ey (V)" <- w1383
                  n504 = Select(t=w1457, s=w1459, f=w1456) -> (s? t:f=w1458:fxp<+/-,58,25>)
                  "Kzx Output, Kzx*ez (V)" <- w1458
                  n505 = Select(t=w1405, s=w1407, f=w1401) -> (s? t:f=w1403:fxp<+/-,58,25>[])
                  n506 = Select(t=w1519, s=w1529, f=w1511) -> (s? t:f=w1513:fxp<+/-,58,25>[])
                  n507 = Select(t=w1492, s=w1497, f=w1486) -> (s? t:f=w1489:fxp<+/-,58,25>[])
                  n508 = Select(t=w1517, s=w1525, f=w1505) -> (s? t:f=w1509:fxp<+/-,58,25>[])
                  n509 = Select(t=w1413, s=w1414, f=w1411) -> (s? t:f=w1412:fxp<+/-,58,25>[])
                  n510 = Select(t=w1406, s=w1409, f=w1402) -> (s? t:f=w1404:fxp<+/-,58,25>[])
                  n511 = Select(t=w1515, s=w1521, f=w1503) -> (s? t:f=w1507:fxp<+/-,58,25>[])
                  n512 = Select(t=w1366, s=w1369, f=w1363) -> (s? t:f=w1361:fxp<+/-,58,25>[])
                  n513 = Select(t=w1490, s=w1493, f=w1484) -> (s? t:f=w1487:fxp<+/-,58,25>[])
                  n514 = Select(t=w1520, s=w1531, f=w1512) -> (s? t:f=w1514:fxp<+/-,58,25>[])
                  n515 = Select(t=w1425, s=w1427, f=w1422) -> (s? t:f=w1423:fxp<+/-,58,25>[])
                  n516 = Select(t=w1518, s=w1527, f=w1506) -> (s? t:f=w1510:fxp<+/-,58,25>[])
                  n517 = Select(t=w1468, s=w1469, f=w1467) -> (s? t:f=w1466:fxp<+/-,58,25>[])
                  n518 = Select(t=w1418, s=w1419, f=w1416) -> (s? t:f=w1417:fxp<+/-,58,25>[])
                  n519 = Select(t=w1491, s=w1495, f=w1485) -> (s? t:f=w1488:fxp<+/-,58,25>[])
                  n520 = Select(t=w1516, s=w1523, f=w1504) -> (s? t:f=w1508:fxp<+/-,58,25>[])
                  n521 = Select(t=w1472, s=w1474, f=w1471) -> (s? t:f=w1473:fxp<+/-,58,25>[])
                  n522 = Select(t=w1396, s=w1399, f=w1394) -> (s? t:f=w1392:fxp<+/-,58,25>[])
                  n523 = Select(t=w1395, s=w1397, f=w1393) -> (s? t:f=w1391:fxp<+/-,58,25>[])
                  n524 = Select(t=w1463, s=w1464, f=w1462) -> (s? t:f=w1461:fxp<+/-,58,25>[])
                  n525 = Select(t=w1365, s=w1367, f=w1362) -> (s? t:f=w1360:fxp<+/-,58,25>[])
                  n526 = Select(t=w1426, s=w1429, f=w1421) -> (s? t:f=w1424:fxp<+/-,58,25>[])
                  n527 = Select(t=w1447, s=w1449, f=w1446) -> (s? t:f=w1448:fxp<+/-,58,25>[])
                  n528 = Select(t=w1443, s=w1444, f=w1441) -> (s? t:f=w1442:fxp<+/-,58,25>[])
                  n529 = Select(t=w1376, s=w1379, f=w1372) -> (s? t:f=w1374:fxp<+/-,58,25>[])
                  n530 = Select(t=w1375, s=w1377, f=w1371) -> (s? t:f=w1373:fxp<+/-,58,25>[])
                  n531 = Select(t=w1453, s=w1454, f=w1451) -> (s? t:f=w1452:fxp<+/-,58,25>[])
                }
              }
            }
            n532 = Add(x=w770, y=w771) -> (x+y=w772:fxp<+/-,59,26>)
            n533 = Add(x=w749, y=w750) -> (x+y=w751:fxp<+/-,59,26>)
            n534 = Add(x=w782, y=w783) -> (x+y=w781:fxp<+/-,59,26>)
            n535 = Add(x=w769, y=w772) -> (x+y=w768:fxp<+/-,60,27>)
            n536 = Add(x=w748, y=w751) -> (x+y=w747:fxp<+/-,60,27>)
            n537 = Add(x=w780, y=w781) -> (x+y=w779:fxp<+/-,60,27>)
            n538 = Multiply(x=w747, y="Scaling mV to V") -> (x*y=w820:fxp<+/-,64,37>)
            n539 = Multiply(x=w779, y="Scaling mV to V") -> (x*y=w819:fxp<+/-,64,37>)
            n540 = Multiply(x=w768, y="Scaling mV to V") -> (x*y=w798:fxp<+/-,64,37>)
            n541 = To Fixed-Point(fixed-point type=w790, number=w819) -> (fixed-point=w821:fxp<+/-,58,25>)
            n542 = To Fixed-Point(fixed-point type=w790, number=w798) -> (fixed-point=w796:fxp<+/-,58,25>)
            n543 = To Fixed-Point(fixed-point type=w790, number=w820) -> (fixed-point=w797:fxp<+/-,58,25>)
          }
        }
        n544 = To Fixed-Point(fixed-point type=w664, number=w668) -> (fixed-point=w667:fxp<+/-,20,5>)
        n545 = To Fixed-Point(fixed-point type=w664, number=w688) -> (fixed-point=w666:fxp<+/-,20,5>)
        n546 = To Fixed-Point(fixed-point type=w664, number=w687) -> (fixed-point=w665:fxp<+/-,20,5>)
        n547 = call "measure_loop_rate_FPGA.vi"() -> ("Loop Rate (Ticks)"=→"Measured Controller Time Period (Ticks)":u32)  [unwired: 11 in]
        n548 = In Range and Coerce(upper limit="Controller Output Upper Limit", x=w667, lower limit="Controller Output Lower Limit") -> (coerced(x)=→"PI X-Stage Input (V)":fxp<+/-,20,5>, In Range?=→"X-Stage Input In Range?":bool)
        n549 = In Range and Coerce(upper limit="Controller Output Upper Limit", x=w666, lower limit="Controller Output Lower Limit") -> (coerced(x)=→"PI Y-Stage Input (V)":fxp<+/-,20,5>, In Range?=→"Y-Stage Input In Range?":bool)
        n550 = In Range and Coerce(upper limit="Controller Output Upper Limit", x=w665, lower limit="Controller Output Lower Limit") -> (coerced(x)=→"PI Z-Stage Input (V)":fxp<+/-,20,5>, In Range?=→"Z-Stage Input In Range?":bool)
        n551 = local read "stop case"() -> (w699:bool)
      }
      n552 = timed-loop {
        timing: w29 -> [_]
        timing-out: [_] -> w28
        tunnel: [w574] -> w22
        shift-right: [w582] -> _
        shift-left: _ -> [w488]
        shift-right: [w581] -> _
        shift-left: _ -> [w580]
        shift-right: [w579] -> _
        shift-left: w15 -> [w578]
        shift-right: [w577] -> _
        shift-left: u32 0 ("Tick Count(Ticks)") -> [w576]
        tunnel: [w575] -> w27
        shift-right: [w562] -> _
        shift-left: _ -> [w560]
        shift-right: [w561] -> _
        shift-left: _ -> [w559]
        shift-right: [w556] -> _
        shift-left: w15 -> [w555]
        shift-right: [w543] -> _
        shift-left: _ -> [w541]
        shift-right: [w542] -> _
        shift-left: _ -> [w540]
        shift-right: [w539] -> _
        shift-left: w15 -> [w538]
        shift-right: [w526] -> _
        shift-left: _ -> [w523]
        shift-right: [w525] -> _
        shift-left: _ -> [w524]
        shift-right: [w522] -> _
        shift-left: w15 -> [w521]
        shift-right: [w509] -> _
        shift-left: _ -> [w506]
        shift-right: [w508] -> _
        shift-left: _ -> [w507]
        shift-right: [w505] -> _
        shift-left: w15 -> [w504]
        tunnel: [w491] -> _
        shift-right: [w492] -> _
        shift-left: _ -> [w490]
        shift-right: [w491] -> _
        shift-left: _ -> [w489]
        shift-right: [w487] -> _
        shift-left: w15 -> [w486]
        stop <- w557 stop-if-true
        w485 = FALSE ("value")
        n553 = xnode "FPGA I/O Node"() -> ("error out"=w574:errorcluster, "Mod4/DIO0"=w582:bool, "Mod4/DIO1"=w581:bool, "Mod4/DIO2"=w526:bool, "Mod4/DIO3"=w525:bool, "Mod5/DIO0"=w562:bool, "Mod5/DIO1"=w561:bool, "Mod5/DIO2"=w509:bool, "Mod5/DIO3"=w508:bool, "Mod6/DIO0"=w543:bool, "Mod6/DIO1"=w542:bool, "Mod6/DIO2"=w492:bool, "Mod6/DIO3"=w491:bool)  [unwired: 13 in, 12 out]
        "Mod4/DIO0" <- w582
        "Mod4/DIO1" <- w581
        "Mod5/DIO0" <- w562
        "Mod5/DIO1" <- w561
        "Mod6/DIO0" <- w543
        "Mod6/DIO1" <- w542
        "Mod4/DIO2" <- w526
        "Mod4/DIO3" <- w525
        "Mod5/DIO2" <- w509
        "Mod5/DIO3" <- w508
        "Mod6/DIO2" <- w492
        "Mod6/DIO3" <- w491
        n554 = Exclusive Or(1:w489, 2:w492) -> (0:w493:bool)
        n555 = Exclusive Or(1:w540, 2:w543) -> (0:w544:bool)
        n556 = Exclusive Or(1:w559, 2:w562) -> (0:w563:bool)
        n557 = Exclusive Or(1:w507, 2:w509) -> (0:w510:bool)
        n558 = call "Tick Count"() -> ("Tick Count(Ticks)"=w577:u32)
        n559 = Exclusive Or(1:w580, 2:w582) -> (0:w583:bool)
        n560 = Exclusive Or(1:w524, 2:w526) -> (0:w527:bool)
        n561 = Select(t=0, s="Reset Sample Z", f=w486) -> (s? t:f=w502:i32)
        n562 = Select(t=0, s="Reset Optics Z", f=w538) -> (s? t:f=w553:i32)
        n563 = Select(t=0, s="Reset Optics Y", f=w555) -> (s? t:f=w572:i32)
        n564 = Exclusive Or(1:w489, 2:w491) -> (0:w499:bool)
        n565 = Exclusive Or(1:w540, 2:w542) -> (0:w550:bool)
        n566 = Exclusive Or(1:w559, 2:w561) -> (0:w569:bool)
        n567 = Select(t=0, s="Reset Sample Y", f=w504) -> (s? t:f=w519:i32)
        n568 = Exclusive Or(1:w507, 2:w508) -> (0:w516:bool)
        n569 = Exclusive Or(1:w490, 2:w492) -> (0:w498:bool)
        n570 = Exclusive Or(1:w541, 2:w543) -> (0:w549:bool)
        n571 = Exclusive Or(1:w560, 2:w562) -> (0:w568:bool)
        n572 = Select(t=1 ("x"), s=w493, f=-1 ("x")) -> (s? t:f=w495:i32)
        n573 = Select(t=1 ("x"), s=w544, f=-1 ("x")) -> (s? t:f=w546:i32)
        n574 = Select(t=1 ("x"), s=w563, f=-1 ("x")) -> (s? t:f=w565:i32)
        n575 = Exclusive Or(1:w506, 2:w509) -> (0:w515:bool)
        n576 = Subtract(x=w577, y=w576) -> (x-y=w575:u32)
        n577 = Select(t=0, s="Reset Optics X", f=w578) -> (s? t:f=w592:i32)
        n578 = Select(t=1 ("x"), s=w510, f=-1 ("x")) -> (s? t:f=w512:i32)
        n579 = Select(t=0, s="Reset Sample X", f=w521) -> (s? t:f=w536:i32)
        n580 = Exclusive Or(1:w580, 2:w581) -> (0:w589:bool)
        n581 = Exclusive Or(1:w524, 2:w525) -> (0:w533:bool)
        n582 = Or(x=w498, y=w499) -> (x .or. y?=w497:bool)
        n583 = Or(x=w549, y=w550) -> (x .or. y?=w548:bool)
        n584 = Or(x=w568, y=w569) -> (x .or. y?=w567:bool)
        n585 = Exclusive Or(1:w488, 2:w582) -> (0:w588:bool)
        n586 = Exclusive Or(1:w523, 2:w526) -> (0:w532:bool)
        n587 = Or(x=w515, y=w516) -> (x .or. y?=w514:bool)
        n588 = Select(t=1 ("x"), s=w583, f=-1 ("x")) -> (s? t:f=w585:i32)
        n589 = Select(t=1 ("x"), s=w527, f=-1 ("x")) -> (s? t:f=w529:i32)
        n590 = Or(x=w588, y=w589) -> (x .or. y?=w587:bool)
        n591 = Or(x=w532, y=w533) -> (x .or. y?=w531:bool)
        n592 = Add(x=w495, y=w502) -> (x+y=w503:i32)
        n593 = Add(x=w546, y=w553) -> (x+y=w554:i32)
        n594 = Add(x=w565, y=w572) -> (x+y=w573:i32)
        n595 = Add(x=w512, y=w519) -> (x+y=w520:i32)
        n596 = Select(t=w503, s=w497, f=w502) -> (s? t:f=w487:i32)
        "32 bit Count Sample  Z" <- w487
        n597 = Select(t=w554, s=w548, f=w553) -> (s? t:f=w539:i32)
        "32 bit Count Optics  Z" <- w539
        n598 = Select(t=w573, s=w567, f=w572) -> (s? t:f=w556:i32)
        "32 bit Count Optics  Y" <- w556
        n599 = Add(x=w585, y=w592) -> (x+y=w593:i32)
        n600 = Add(x=w529, y=w536) -> (x+y=w537:i32)
        n601 = Select(t=w520, s=w514, f=w519) -> (s? t:f=w505:i32)
        "32 bit Count Sample  Y" <- w505
        n602 = local read "stop case"() -> (w558:bool)
        n603 = Select(t=w593, s=w587, f=w592) -> (s? t:f=w579:i32)
        "32 bit Count Optics X" <- w579
        n604 = Select(t=w537, s=w531, f=w536) -> (s? t:f=w522:i32)
        "32 bit Count Sample X" <- w522
        n605 = Compound Arithmetic op=OR(w485, w485, w485, w558) -> (w557:bool)
      }
      "Measured Counter Time Period (Ticks)" <- w27
      n606 = while {
        stop <- w31 stop-if-true
        n607 = local read "DT Frequency (periods/tick)"() -> (w35:fxp<+,32,0>)
        n608 = local read "DT Phase Offset (periods)"() -> (w34:fxp<+,32,0>)
        n609 = local read "DT Duty Cycle (periods)"() -> (w33:fxp<+,32,0>)
        n610 = local read "DT Reset"() -> (w32:bool)
        n611 = call "Square Wave Generator2"("frequency (periods/tick)"=w35, "reset"=w32, "phase offset (periods)"=w34, "duty cycle (periods)"=w33) -> ("square wave out"=w42:i16)  [unwired: 11 in]
        n612 = call "Loop Timer11"("Count(uSec)"="Data Trigger Time Period (uSec)") -> ()  [unwired: 1 out]
        n613 = call "measure_loop_rate_FPGA.vi"() -> ("Loop Rate (Ticks)"=→"Measured Data Trigger Time Period (Ticks)":u32)  [unwired: 11 in]
        n614 = Divide(x=w42, y=i16 32767) -> (x/y=w38:fxp<+/-,41,18>)
        n615 = To Fixed-Point(fixed-point type=fxp<+/-,58,25> 0.0, number=w38) -> (fixed-point=→"Trigger for Data":fxp<+/-,58,25>)
        n616 = local read "stop case"() -> (w31:bool)
      }
      n617 = node-c288(w28) -> (w23:errorcluster)
      n618 = while {
        tunnel: [w287] -> w18
        stop <- w292 stop-if-true
        n619 = local read "Detector Trigger (V)"() -> (w288:fxp<+/-,20,5>)
        n620 = call "Loop Timer8"("Count(uSec)"="Detector Trigger Time Period (uSec)") -> ()  [unwired: 1 out]
        n621 = call "measure_loop_rate_FPGA.vi"() -> ("Loop Rate (Ticks)"=→"Measured Detector Trigger Time Period (Ticks)":u32)  [unwired: 11 in]
        n622 = xnode "FPGA I/O Node"("I/O Item"=w288, "FPGA I/O In"=refnum<k21> "Mod8/AO3") -> ("error out"=w287:errorcluster)  [unwired: 1 in, 1 out]
        n623 = local read "stop case"() -> (w292:bool)
      }
      n624 = Merge Errors "Merge Errors"(w18, w20, w19, w23, w22, w24) -> (w30:errorcluster)
    }
    frame Error {
      n625 = local write "stop case"(TRUE ("stop case")) -> ()
      n626 = xnode "FPGA I/O Node"("Mod3/Stop"=TRUE ("I/O Item")) -> ()  [unwired: 1 in, 1 out]
    }
  }
  "error out (FPGA)" <- w2
